vi "Setting_Screen.vi"(8 "error in (no error)":errorcluster) -> (0 "error in (out)":errorcluster)   [LabVIEW 2024, in "Setting_Screen.lvlib"]
doc: "This template is for the Queued Message Handler design pattern.\n\nThe Event Handling Loop generates messages based on user interface actions.\n\nThe Message Handling Loop processes messages generated by the Event Handling Loop, or by other messages. The messages are string values, so new messages can be added easily to the Message Cases case structure in the Message Handling Loop. Each message cluster can also provide an optional value for Message Data, which is a variant that can be converted to whatever message-specific data is required."
uses:
  Setting_Screen.lvlib
  support/Steptab.ctl
  support/PS_WRITE.ctl
  support/PS_set.ctl
  support/DMM_CONFIG.ctl
  support/READ_DATAS.ctl
  support/READ_EQP.ctl
  support/READ_PARA.ctl
  support/Relay_Channel_Array.ctl
  support/Common_plc_DOs.ctl
  support/DAQ_Config.ctl
  PCANusb_DTU/support/CAN_MSGs.ctl
  PCANusb_DTU/support/CAN_Frames_ctrl.ctl
  PCANusb_DTU/support/Framing datas.ctl
  PCANusb_DTU/support/CAN_Read.ctl
  support/Camera.ctl
  MCU_Flashing/support/MCU_ctrl.ctl
  support/Neoway ctl.ctl
  support/SSL.ctl
  controls/Setting_Screen UI Data.ctl
  support/ScriptDetails.ctl
  support/CurrentStep.ctl
  support/StepType.ctl
  PrivateControls/Setting_Screen_FGV_Queue_Control.ctl
  <vilib>/Utility/error.llb/Error Cluster From Error Code.vi
  <vilib>/ErrorRing/Error Ring.xnode
  support/Message Queue/Setting_Screen_Message Queue.lvlib
  support/User Event - Stop/Setting_Screen_User Event - Stop.lvlib
  Launcher/Launcher_DTU.lvlib
  Launcher/MainLauncher.vi
  PCANusb_DTU/PCANusb_DTU.lvlib
  MCU_Flashing/MCU_Flashing.lvlib
panel:
  out "Step no.":i16
  in  "New Step Name":string
  in  "Configurations:":string(combo)
  in  "Rename Step":bool
  in  "Instr.":bool
  in  "STEP_DOWN":bool
  in  "STEP_UP":bool
  in  "ADD NEXT SCRIPT":bool
  in  "SaveAs Name:":string
  in  "New_Config_name":string
  in  "New Config":bool
  in  "Save As":bool
  in  "Save":bool
  in  "UpdateStep":bool
  in  "Delete Step":bool
  in  "Delete Script":bool
  in  "Add Step":bool
  in  "Add Script":bool
  in  "Step Name":string
  in  "Script Name":string
  in  "Tab Control":T1
  in  "Set_Channel_Relay":T2 {"Relay_CH_Array"."OUTPUT_Relay_Channels" items=["CONN_SUPPLY_%d_FCT", "HB_CONN_%d_FCT", "L_IND_CONN_%d_FCT", "R_IND_CONN_%d_FCT", "SW1_%d_FCT", "SW2_%d_FCT", "CAN_H_%d_FCT", "CAN_L_%d_FCT", "CYLINDER_ON/OFF_%d_FCT", "SPARE_1_%d_FCT", "SPARE_2_%d_FCT", "Tower Red", "Tower Amber", "Tower Green", "Tower Buzzer", "SLIMRELAY_DUT_%d_FCT", "GND_DMM_%d_EOL", "CAN_H_RES_%d_EOL", "CAN_L_RES_%d_EOL", "L_IND_RES_%d_EOL", "R_IND_RES_%d_EOL", "HB_CONN_DMM_%d_EOL", "14V_RES_%d_EOL", "CAN_L_(DMM-)_%d_EOL", "CAN_H_%d_EOL", "CAN_L_%d_EOL", "14V_%d_EOL", "GND_%d_EOL", "HB_CONN_%d_EOL", "L_IND_%d_EOL", "R_IND_%d_EOL", "CYLINDER_DUT_%d_EOL", "CYL_PB_1_%d_EOL", "CYL_PB_2_%d_EOL", "DUT_PASS_%d_EOL", "DUT_FAIL_%d_EOL", "SPARE1_%d_EOL", "Tower Red_EOL", "Tower Amber_EOL", "Tower Green_EOL", "Tower Buzzer_EOL"]}
  in  "PS_Write":T4 {"Set_parameter" items=["Set_Voltage", "Set_current", "Output"]}
  in  "READ_DATAS":T6 {"PARAMETER" items=["SET_VOLTAGE", "SET_CURRENT", "OUTPUT VOLTAGE", "OUTPUT CURRENT", "RESISTANCE", "OUTPUT POWER", "CAMERA", "SSL_Check"]; "EQUIPMENT" items=["POWER SUPPLY", "DMM", "DAQ", "CAMERA"]}
  in  "DMM_CONFIG":T9 {"CONFIG PARAMETER" items=["VOLTAGE", "CURRENT", "RESISTANCE", "POWER"]}
  in  "DAQ_Config":T10 {"Function" items=["Voltage DC", "Voltage AC", "Current DC", "Current AC", "Resistance", "4-wire Resistance", "Diode", "Capacitance", "Temperature", "Continuity", "Frequency", "Period", "Voltage Ratio", "Digitize Voltage", "Digitize Current"]; "SELECT SLOT" items=["Slot 1", "Slot 2"]; "SELECT Card" items=["7708", "7700"]}
  in  "CAN_MSGs_Write":T11={"Scaling Factor"=1, "Physical value"=0.0, "CAN_Frames"={"CAN_ID"=0, "MSGTYPE"=128, "Payload"=[], "Length"=0}, "Offset value"=0.0, "Framing datas"=[], "CAN_Frame Enable"=FALSE, "Add Signal"=FALSE, "Delete Signal"=FALSE, "Signal Values"=[], "Time(ms)"=0.0, "Repetition"=FALSE, "Delay"=FALSE, "Delay time"=0.0} {"CAN_Frames"."Payload" format="%.0x"; "CAN_Frames"."MSGTYPE" items=["STATUS"=128, "EXTENDED"=2, "RTR"=1, "DATA MSG"=0]; "CAN_Frames"."CAN_ID" format="%.0x"}
  in  "CAN_Read":T14 {"SUB-SERVICE ID" format="%.0x"; "SERVICE ID" format="%.0x"; "CANID" format="%.0x"; "ReadPayload" format="%.0x"}
  in  "Camera":T15
  in  "Noeway_Flashing":T16
  in  "MCU Flashing":T17
  in  "SSL":T18
  in  "Script_Tree":string(tree)
  out "queue name 2":string
  out "queue name":string
  in  "New Step":bool
  in  "New Script":bool
  in  "Exit":bool
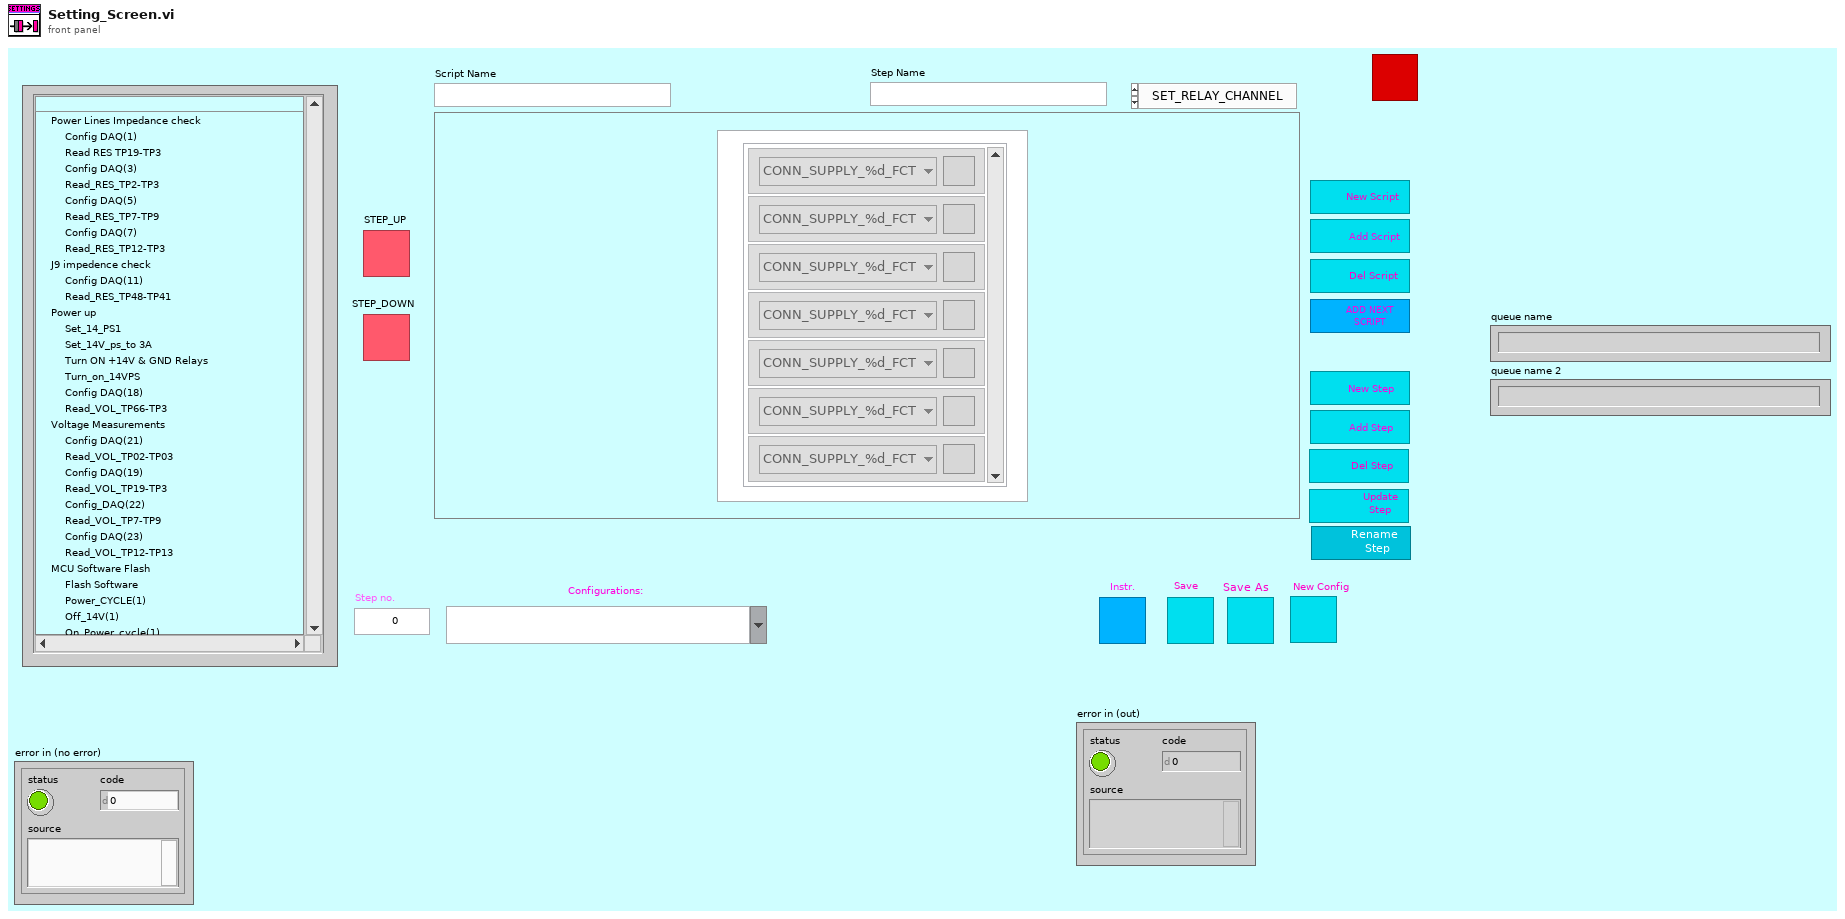
[diagram p1: front panel]
types:
  T1 = typedef "Setting_Screen.lvlib/Steptab.ctl" = enum32{"SET_RELAY_CHANNEL", "PS_WRITE", "READ_DATA", "DMM_CONFIG", "DAQ_Config", "CAN_Write", "CAN_Read", "Camera", "Noeway_Flashing", "MCU_Flashing", "SSL_Certification"}
  T2 = typedef "Setting_Screen.lvlib/Relay_Channel_Array.ctl" = cluster{"Relay_CH_Array":cluster{"OUTPUT_Relay_Channels":T3, "On/Off":bool}[]}
  T3 = typedef "Setting_Screen.lvlib/Common_plc_DOs.ctl" = u16
  T4 = typedef "Setting_Screen.lvlib/PS_WRITE.ctl" = cluster{"Set_parameter":T5, "VOLTAGE":string, "CURRENT":string, "OUTPUT":bool, "Delay":bool, "Delay time":dbl}
  T5 = typedef "Setting_Screen.lvlib/PS_set.ctl" = u16
  T6 = typedef "Setting_Screen.lvlib/READ_DATAS.ctl" = cluster{"EQUIPMENT":T7, "PARAMETER":T8, "LSL":dbl, "USL":dbl, "RESULT":string, "UNIT":string, "Delay":bool, "Delay time":dbl}
  T7 = typedef "Setting_Screen.lvlib/READ_EQP.ctl" = u16
  T8 = typedef "Setting_Screen.lvlib/READ_PARA.ctl" = u16
  T9 = typedef "Setting_Screen.lvlib/DMM_CONFIG.ctl" = cluster{"CONFIG PARAMETER":u16, "AUTO RANGE":bool, "RANGE":string, "Delay":bool, "Delay time":dbl}
  T10 = typedef "Setting_Screen.lvlib/DAQ_Config.ctl" = cluster{"AUTO RANGE":bool, "CHANNEL LIST":string, "SELECT Card":u16, "SELECT SLOT":u16, "Function":i32}
  T11 = typedef "PCANusb_DTU.lvlib/CAN_MSGs.ctl" = cluster{"Scaling Factor":u16, "Physical value":dbl, "CAN_Frames":T12, "Offset value":dbl, "Framing datas":T13[], "CAN_Frame Enable":bool, "Add Signal":bool, "Delete Signal":bool, "Signal Values":dbl[], "Time(ms)":dbl, "Repetition":bool, "Delay":bool, "Delay time":dbl}
  T12 = typedef "PCANusb_DTU.lvlib/CAN_Frames_ctrl.ctl" = cluster{"CAN_ID":u32, "MSGTYPE":u8, "Payload":u8[], "Length":u8}
  T13 = typedef "PCANusb_DTU.lvlib/Framing datas.ctl" = cluster{"Signal name":string, "Start Bit":u8, "Length":u8, "Value":u16}
  T14 = typedef "PCANusb_DTU.lvlib/CAN_Read.ctl" = cluster{"Database":refnum<k21>, "Signal":refnum<k21>, "BYTES":u32[], "ReadPayload":u8[], "String_Data":string, "ReadValue":dbl, "CANID":u32, "SERVICE ID":u32, "SUB-SERVICE ID":u32, "DELAY ":bool, "Delay time(ms)":dbl}
  T15 = typedef "Setting_Screen.lvlib/Camera.ctl" = cluster{"Trigger":bool, "Prog No.":string, "Delay":bool, "Delay time":dbl, "Storage":string, "Col no.":string, "Row no.":string}
  T16 = typedef "Neoway ctl.ctl" = cluster{"Neoway_Firmware":path, "RESULT STRING":string, "Delay":bool, "Delay time":dbl}
  T17 = typedef "MCU_Flashing.lvlib/MCU_ctrl.ctl" = cluster{"Result Path":path, "Result":string}
  T18 = typedef "SSL.ctl" = cluster{"SSL_EXE":path, "RESULT STRING":string, "Delay":bool, "Delay time":dbl}
  T19 = typedef "Setting_Screen.lvlib/Setting_Screen_FGV_Queue_Control.ctl" = enum16{"Release", "Get", "Set"}
  T20 = typedef "Setting_Screen.lvlib/Setting_Screen UI Data.ctl" = cluster{"Script_Tree":refnum<vi>, "Scripts":T21[], "ScriptDetails":T21, "Current Step":T22, "ScriptName":string, "StepName":string, "Children Symbols":i32[][], "Parrent Symbol":i32[], "Configurations:":string, "Config":string, "Scriptno.":i32, "PS_Write":T4, "DMM_CONFIG":T9, "READ_DATAS":T6, "Set_Channel_Relay":T2, "DAQ_Config":T10, "CAN_MSGs_Write":T11, "CAN_Read":T14, "Camera":T15, "Tab Control":refnum<vi>, "MCU Flashing":T17, "Noeway_Flashing":T16, "SSL":T18}
  T21 = typedef "Setting_Screen.lvlib/ScriptDetails.ctl" = cluster{"Script Name":string, "Steps":T22[]}
  T22 = typedef "Setting_Screen.lvlib/CurrentStep.ctl" = cluster{"StepName":string, "StepDetails":string, "Type":T23}
  T23 = typedef "Setting_Screen.lvlib/StepType.ctl" = enum16{"RELAY_CHANNEL_WRITE", "PS_WRITE", "READ_DATA", "DMM_CONFIG", "DAQ_CONFIG", "PCAN_Read", "PCAN_Write", "Camera", "MCU_Flashing", "Noeway_Flashing", "SSL_Certification"}
  T24 = typedef "Setting_Screen.lvlib/Setting_Screen_Message Queue.lvlib/Setting_ScreenAll Message Queues.ctl" = cluster{"UI":refnum<queue>, "QSM":refnum<queue>}
  T25 = enum16{"Next Item", "Previous Item", "Get Child", "Get Parent", "Get Path"}
  T26 = enum16{"Read", "Write", "All_sections", "All_values", "Remove key&section"}
  T27 = enum32{"Invalid", "Standard", "Closed", "Hidden", "Minimized", "Maximized"}
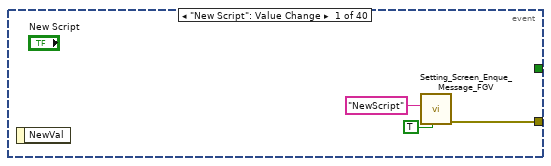
[diagram p3: hidden frame]
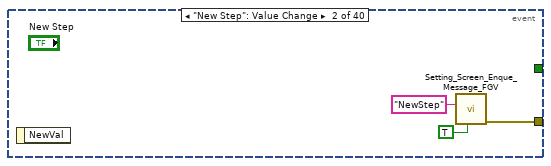
[diagram p4: hidden frame]
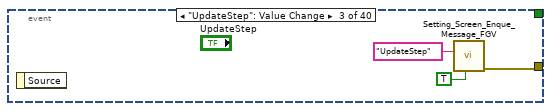
[diagram p5: hidden frame]
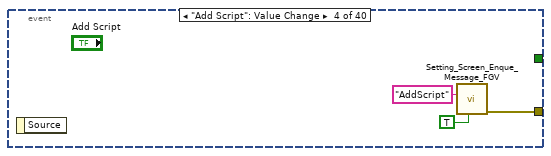
[diagram p6: hidden frame]
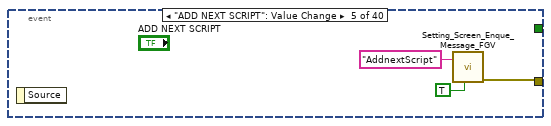
[diagram p7: hidden frame]
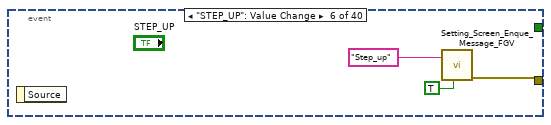
[diagram p8: hidden frame]
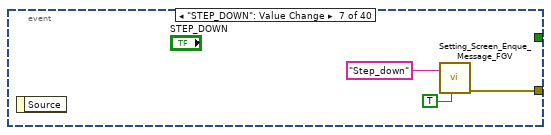
[diagram p9: hidden frame]
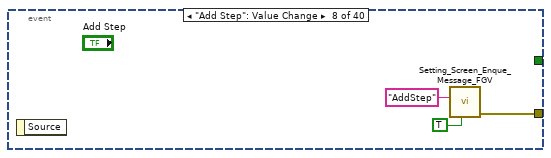
[diagram p10: hidden frame]
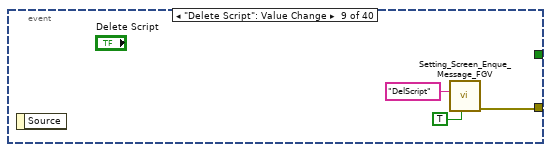
[diagram p11: hidden frame]
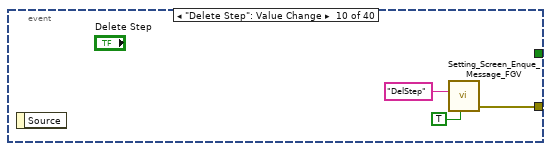
[diagram p12: hidden frame]
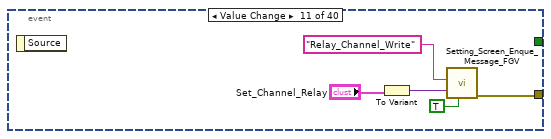
[diagram p13: hidden frame]
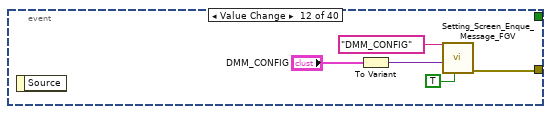
[diagram p14: hidden frame]
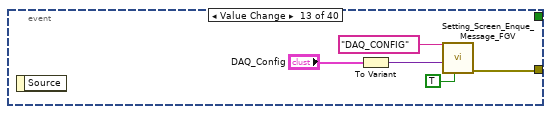
[diagram p15: hidden frame]
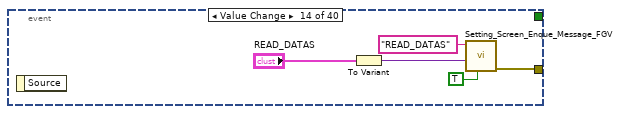
[diagram p16: hidden frame]
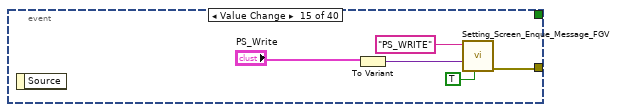
[diagram p17: hidden frame]
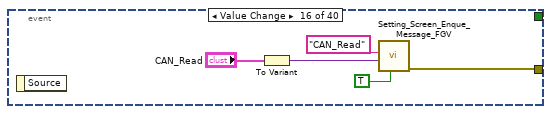
[diagram p18: hidden frame]
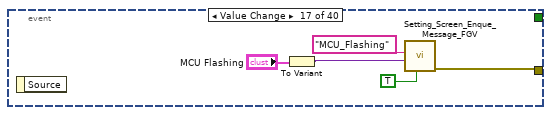
[diagram p19: hidden frame]
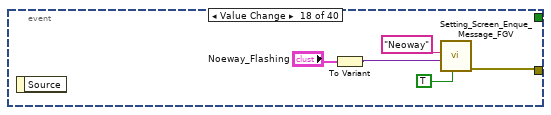
[diagram p20: hidden frame]
diagram:
  (unwired) 40
  (unwired) "\u0000\u0000\u0000\u0000\u0000\u0000\u0000\u000f\u0000\u0000\u0000\u0000\u0000\u0000\u0000\u0001\u0000\u0000\u0000\u0000\u0000\u0000\u0000\u0000\u0000\u0000\u0000\u0000\u0000#Signal connector J9 impedence check\u0000\u0000\u0000\u0016\u0000\u0000\u0000\u000eConfig_DMM_RES\u0000\u0000\u0000\u0010\u0000\u0002\u0001\u0000\u0000\u0000\u0000\u0000\u0000\u0000\u0000\u0000\u0000\u0000\u0000\u0000\u0000\u0003\u0000\u0000\u0000\u001aTurn ON CAN_H & GND Relays\u0000\u0000\u0000\n\u0000\u0000\u0000\u0002\u0000\u0010\u0001\u0000\u0011\u0001\u0000\u0000\u0000\u0000\u0000\u0015Read RES CAN_H to GND\u0000\u0000\u0000)\u0000\u0001\u0000\u0004?ð\u0000\u0000\u0000\u0000\u0000\u0000@$\u0000\u0000\u0000\u0000\u0000\u0000\u0000\u0000\u0000\u0000\u0000\u0000\u0000\u0004Mohm\u0000\u0000\u0000\u0000\u0000\u0000\u0000\u0000\u0000\u0000\u0002\u0000\u0000\u0000\u0015Turn OFF CAN _H Relay\u0000\u0000\u0000\u0007\u0000\u0000\u0000\u0001\u0000\u0011\u0000\u0000\u0000\u0000\u0000\u0000\u0013Turn ON CAN_L Relay\u0000\u0000\u0000\u0007\u0000\u0000\u0000\u0001\u0000\u0012\u0001\u0000\u0000\u0000\u0000\u0000\u0015Read RES CAN_L to GND\u0000\u0000\u0000)\u0000\u0001\u0000\u0004?ð\u0000\u0000\u0000\u0000\u0000\u0000@$\u0000\u0000\u0000\u0000\u0000\u0000\u0000\u0000\u0000\u0000\u0000\u0000\u0000\u0004Mohm\u0000\u0000\u0000\u0000\u0000\u0000\u0000\u0000\u0000\u0000\u0002\u0000\u0000\u0000\u001bTurn OFF CAN_L & GND Relays\u0000\u0000\u0000\n\u0000\u0000\u0000\u0002\u0000\u0010\u0000\u0000\u0012\u0000\u0000\u0000\u0000\u0000\u0000\u001cTurn ON CAN_H & CAN_L Relays\u0000\u0000\u0000\n\u0000\u0000\u0000\u0002\u0000\u0011\u0001\u0000\u0017\u0001\u0000\u0000\u0000\u0000\u0000\u0016Read RES CAN_H & CAN_L\u0000\u0000\u0000(\u0000\u0001\u0000\u0004@]\u0000\u0000\u0000\u0000\u0000@^\u0000\u0000\u0000\u0000\u0000\u0000\u0000\u0000\u0000\u0000\u0000\u0000\u0003ohm\u0000\u0000\u0000\u0000\u0000\u0000\u0000\u0000\u0000\u0000\u0002\u0000\u0000\u0000\u001dTurn OFF CAN_H & CAN_L Relays\u0000\u0000\u0000\n\u0000\u0000\u0000\u0002\u0000\u0011\u0000\u0000\u0017\u0000\u0000\u0000\u0000\u0000\u0000\u001aTurn ON..." ("data string")
  w20 = T20 {"Script_Tree"=refnum, "Scripts"=[], "ScriptDetails"={"Script Name"="", "Steps"=[]}, "Current Step"={"StepName"="", "StepDetails"="", "Type"=enum."RELAY_CHANNEL_WRITE"}, "ScriptName"="", "StepName"="", "Children Symbols"=[], "Parrent Symbol"=[], "Configurations:"="", "Config"="", "Scriptno."=0, "PS_Write"={"Set_parameter"=0, "VOLTAGE"="", "CURRENT"="", "OUTPUT"=FALSE, "Delay"=FALSE, "Delay time"=0.0}, "DMM_CONFIG"={"CONFIG PARAMETER"=0, "AUTO RANGE"=FALSE, "RANGE"="", "Delay"=FALSE, "Delay time"=0.0}, "READ_DATAS"={"EQUIPMENT"=0, "PARAMETER"=0, "LSL"=0.0, "USL"=0.0, "RESULT"="", "UNIT"="", "Delay"=FALSE, "Delay time"=0.0}, "Set_Channel_Relay"={"Relay_CH_Array"=[]}, "DAQ_Config"={"AUTO RANGE"=FALSE, "CHANNEL LIST"="", "SELECT Card"=0, "SELECT SLOT"=0, "Function"=0}, "CAN_MSGs_Write"={"Scaling Factor"=0, "Physical value"=0.0, "CAN_Frames"={"CAN_ID"=0, "MSGTYPE"=0, "Payload"=[], "Length"=0}, "Offset value"=0.0, "Framing datas"=[], "CAN_Frame Enable"=FALSE, "Add Signal"=FALSE, "Delete Signal"=FALSE, "Signal Values"=[], "Time(ms)"=0.0, "Repetition"=FALSE, "Delay"=FALSE, "Delay time"=0.0}, "CAN_Read"={"Database"="", "Signal"="", "BYTES"=[], "ReadPayload"=[], "String_Data"="", "ReadValue"=0.0, "CANID"=0, "SERVICE ID"=0, "SUB-SERVICE ID"=0, "DELAY "=FALSE, "Delay time(ms)"=0.0}, "Camera"={"Trigger"=FALSE, "Prog No."="", "Delay"=FALSE, "Delay time"=0.0, "Storage"="", "Col no."="", "Row no."=""}, "Tab Control"=refnum, "MCU Flashing"={"Result Path"=path "", "Result"=""}, "Noeway_Flashing"={"Neoway_Firmware"=path "", "RESULT STRING"="", "Delay"=FALSE, "Delay time"=0.0}, "SSL"={"SSL_EXE"=path "", "RESULT STRING"="", "Delay"=FALSE, "Delay time"=0.0}}  # Data Cluster
  # "MCU_Flashing"
  n1 = control-ref of="This VI"() -> (w15:refnum<vi>)
  n2 = call "Setting_Screen_Pre_Loop_Initialization_FGV.vi"("error in (no error)"="error in (no error)", "VI in"=w15) -> ("error out"=w13:errorcluster, "User Event out"=w4:refnum<user-event>)  [unwired: 8 in]
  n3 = call "Create User Event - Stop.vi"("error in (no error)"=w13) -> ("error out"=w8:errorcluster, "User Event - Stop"=w3:refnum<user-event>)  [unwired: 9 in]
  n4 = control-ref of="This VI"() -> (w11:refnum<vi>)
  n5 = register-events(w3, w4) -> (reference out=w18:refnum<event-registration>, error out=w16:errorcluster)  [unwired: 2 in]
  n6 = call "Setting_Screen_Create All Message Queues.vi"("error in (no error)"=w8, "This VI"=w11) -> ("error out"=w27:errorcluster, "Message Queues out"=w26:T24)  [unwired: 8 in]
  n7 = Unbundle By Name(w26) -> ("UI"=w24:refnum<queue>)
  n8 = call "Setting_Screen_Queue_Comm_FGV.vi"("error in (no error)"=w8, "Enum"=Setting_Screen_FGV_Queue_Control."Get") -> ("queue Out"=w6:refnum<queue>)  [unwired: 8 in, 1 out]
  n9 = Get Queue Status(queue=w24) -> (queue out=w10:refnum<queue>, queue name=→"queue name":string)  [unwired: 2 in, 6 out]
  n10 = Get Queue Status(queue=w6) -> (queue name=→"queue name 2":string)  [unwired: 2 in, 7 out]
  n11 = Merge Errors(w16, w27) -> (w17:errorcluster)
  n12 = while {
    tunnel: w10 -> [_]
    shift-right: [w37] -> _
    shift-left: w20 -> [w38]
    tunnel: w4 -> [w35]
    tunnel: w17 -> [w34]
    tunnel: [w29] -> w25
    tunnel: w3 -> [w28]
    stop <- w36 stop-if-true
    # "Message Handling Loop FGV"
    n13 = call "Setting_Screen_Dequeue_Message_FGV.vi"("error in (no error)"=w34) -> ("error out"=w33:errorcluster, "Message Data"=w32:variant, "Message"=w31:string)  [unwired: 8 in]
    n14 = case "Message Cases" shown="\"AddnextScript\"" w31 {
      selector: w31 -> [_ _ _ _ _ _ _ _ _ _ _ _ _ _ _ _ _ _ _ _ _ _ _ _ _ _ _ _ _ _ _ _ _ _ _ _ _ _ _ _ _ _ _ _ _ w918]
      tunnel: w33 -> [w55 w83 w129 w144 w170 w189 w199 w207 w222 w249 w272 w292 w312 w345 w374 w386 w417 w453 w470 w483 w496 w509 w522 w535 w548 w561 w578 w604 w607 w614 w629 w642 w654 w778 w813 w819 w844 w851 w860 w867 w874 w890 w898 w901 w909 _]
      tunnel: [w66 w75 w107 w135 w169 w194 w204 w206 w220 w247 w268 w290 w310 w343 w373 w384 w415 w452 w470 w480 w492 w505 w518 w531 w544 w557 w566 w600 w608 w613 w628 w641 w653 w761 w795 w818 w843 w850 w859 w865 w872 w891 w892 w903 w915 w919] -> w30
      tunnel: w38 -> [w68 w85 w126 w133 w183 w195 w205 w210 w217 w244 w271 w285 w307 w340 w375 w381 w412 w450 w469 w478 w489 w502 w515 w528 w541 w554 w573 w597 w611 w619 w627 w640 w650 w777 w812 w820 w845 w852 w858 w866 w873 w889 w897 w904 w917 w920]
      tunnel: [w67 w85 w118 w139 w175 w187 w197 w210 w216 w243 w270 w284 w306 w338 w375 w380 w411 w444 w468 w481 w493 w506 w519 w532 w545 w558 w575 w601 w609 w617 w626 w639 w649 w758 w792 w820 w840 w852 w858 w862 w869 w889 w897 w904 w917 w920] -> w37
      tunnel: [_ _ _ _ _ _ _ _ _ _ _ _ _ _ _ _ _ _ _ _ _ _ _ _ _ _ _ _ _ _ _ _ _ _ _ _ _ _ _ _ _ _ _ _ TRUE _] -> w36
      tunnel: w32 -> [_ _ w103 w143 _ _ _ _ _ _ _ _ _ w336 _ _ _ _ _ w473 w494 w507 w520 w533 w546 w559 w576 w602 _ _ w624 w637 _ _ w783 _ w841 _ _ w863 w870 _ w896 _ w911 _]
      tunnel: w35 -> [_ _ _ _ _ _ _ _ _ _ _ _ _ _ _ _ _ _ _ _ _ _ _ _ _ _ _ _ _ _ _ _ _ _ _ _ _ _ _ _ _ _ _ _ w914 _]
      tunnel: w28 -> [_ _ _ _ _ _ _ _ _ _ _ _ _ _ _ _ _ _ _ _ _ _ _ _ _ _ _ _ _ _ _ _ _ _ _ _ _ _ _ _ _ _ _ _ w907 _]
      frame "Initialize" {
        w40 = T2 {"Relay_CH_Array"=[{"OUTPUT_Relay_Channels"=0, "On/Off"=FALSE}]}  # Set_Channel_Relay
        w43 = T9 {"CONFIG PARAMETER"=0, "AUTO RANGE"=FALSE, "RANGE"="", "Delay"=FALSE, "Delay time"=0.0}  # DMM_CONFIG
        w44 = T6 {"EQUIPMENT"=0, "PARAMETER"=0, "LSL"=0.0, "USL"=0.0, "RESULT"="", "UNIT"="", "Delay"=FALSE, "Delay time"=0.0}  # READ_DATAS
        w45 = T4 {"Set_parameter"=0, "VOLTAGE"="", "CURRENT"="", "OUTPUT"=FALSE, "Delay"=FALSE, "Delay time"=0.0}  # PS_Write
        w56 = ""
        w60 = ""
        w62 = T22 {"StepName"="", "StepDetails"="", "Type"=enum."RELAY_CHANNEL_WRITE"}  # Current Step
        w63 = T21 {"Script Name"="", "Steps"=[]}  # ScriptDetails
        w64 = T21[] [{"Script Name"="", "Steps"=[{"StepName"="", "StepDetails"="", "Type"=enum."RELAY_CHANNEL_WRITE"}]}]  # Scripts
        # "Initialize"
        n15 = control-ref of="Script_Tree"() -> (w54:refnum<vi>)
        n16 = property on="SaveAs Name:" class="Str"("Visible"=FALSE, "Value"="" ("SaveAs Name:")) -> ()  [unwired: 2 in, 2 out]
        n17 = property on="New Step Name" class="Str"("Visible"=FALSE, "Value"="" ("New Step Name")) -> ()  [unwired: 2 in, 2 out]
        n18 = property class="Tree (strict)"(reference=w54, error in=w55) -> (reference out=w52:refnum<vi>, error out=w53:errorcluster, "All Tags"=w51:string[])
        n19 = property on="New_Config_name" class="Str"("Value"="" ("New_Config_name"), "Visible"=FALSE) -> ()  [unwired: 2 in, 2 out]
        n20 = property on="Configurations:" class="CmbBox"("Strings[]"=string[] [] ("Strings []")) -> ()  [unwired: 2 in, 2 out]
        n21 = for {
          tunnel: w52 -> [w73]
          tunnel: w51 -> [w72] mode=indexing
          shift-right: [w69] -> w50
          shift-left: w53 -> [w74]
          n22 = invoke class="Tree (strict)" method="Edit Tree Items.Delete"(reference=w73, error in=w74, "tag"=w72, "Delete Children"=TRUE ("Delete Children?")) -> (error out=w70:errorcluster)  [unwired: 1 in, 4 out]
          n23 = call <vilib>:"Clear Errors.vi"("error in (no error)"=w70) -> ("error out"=w69:errorcluster)  [unwired: 5 in, 1 out]
        }
        n24 = control-ref of="Script_Tree"() -> (w61:refnum<vi>)
        n25 = control-ref of="Tab Control"() -> (w39:refnum<vi>)
        n26 = Bundle By Name(cluster=w68, "DMM_CONFIG"=w43, "READ_DATAS"=w44, "Scriptno."=0, "Script_Tree"=w61, "Tab Control"=w39, "PS_Write"=w45, "Set_Channel_Relay"=w40, "Scripts"=w64, "ScriptDetails"=w63, "Current Step"=w62, "ScriptName"=w60, "StepName"=w60, "Config"=w60, "Configurations:"="") -> (w67:T20)
        n27 = local write "Script_Tree"(w56) -> ()
        n28 = property class="Tree (strict)"(reference=w61, "Value"=w56) -> ()  [unwired: 1 in, 2 out]
        n29 = call "Setting_Screen_Enque_Message_FGV.vi"("error in (no error)"=w50, "Message"="ReadConfig") -> ("error out"=w66:errorcluster)  [unwired: 9 in]
      }
      frame "ReadConfig" {
        n30 = call "Specify_Path.vi"("Path_Enum"=enum16{"Find_Path", "Get_Path"}."Get_Path", "error in (no error)"=w83) -> ("Settings"=w78:path, "error out"=w82:errorcluster)  [unwired: 6 in, 6 out]
        n31 = List Folder(path=w78, error in=w82) -> (filenames=w79:string[], error out=w81:errorcluster)  [unwired: 2 in, 2 out]
        n32 = Empty Array?(array=w79) -> (empty?=w80:bool)
        n33 = case shown="False" w80 {
          tunnel: w81 -> [w90 w96]
          tunnel: [w90 w96] -> w76
          tunnel: w79 -> [w88 _]
          tunnel: w78 -> [w89 _]
          frame False {
            n34 = for {
              tunnel: w89 -> [w93]
              tunnel: w88 -> [w92] mode=indexing
              tunnel: [w91] -> w87 mode=indexing
              n35 = Build Path(base path=w93, name or relative path=w92) -> (appended path=w94:path)
              n36 = call <vilib>:"Get File Extension.vi"("file"=w94) -> ("filename without extension"=w91:string)  [unwired: 6 in, 4 out]
            }
            n37 = property on="Configurations:" class="CmbBox"("Strings[]"=w87, "Value"="" ("Configurations:")) -> ()  [unwired: 2 in, 2 out]
          }
          frame True {
            n38 = property on="New_Config_name" class="Str"("Visible"=TRUE) -> ()  [unwired: 2 in, 2 out]
          }
        }
        n39 = call "Setting_Screen_Enque_Message_FGV.vi"("error in (no error)"=w76, "Message"="Update Display") -> ("error out"=w75:errorcluster)  [unwired: 9 in]
      }
      frame "ReadSelected" {
        n40 = Variant To Data(error in=w129, type="" ("Configurations:"), Variant=w103) -> (data=w99:string, error out=w104:errorcluster)
        n41 = Unbundle By Name(w126) -> ("Configurations:"=w100:string)
        n42 = call <vilib>:"Clear Errors.vi"("error in (no error)"=w104) -> ("error out"=w98:errorcluster)  [unwired: 5 in, 1 out]
        n43 = Empty String/Path?(string/path=w99) -> (empty?=w101:bool)
        n44 = call "Specify_Path.vi"("Path_Enum"=enum16{"Find_Path", "Get_Path"}."Get_Path", "error in (no error)"=w98) -> ("Settings"=w105:path, "error out"=w128:errorcluster)  [unwired: 6 in, 6 out]
        n45 = Select(t=w100, s=w101, f=w99) -> (s? t:f=w97:string)
        n46 = Concatenate Strings(w97, ".bin" ("string")) -> (w125:string)
        n47 = Build Path(base path=w105, name or relative path=w125) -> (appended path=w122:path)
        n48 = call "BIN_File.vi"("Enum"=enum16{"Read", "Write"}."Read", "error in"=w128, "Path"=w122) -> ("error out"=w123:errorcluster, "data out"=w120:string)  [unwired: 7 in]
        n49 = Unflatten From String(type=T20 {"Script_Tree"=refnum, "Scripts"=[], "ScriptDetails"={"Script Name"="", "Steps"=[]}, "Current Step"={"StepName"="", "StepDetails"="", "Type"=enum."RELAY_CHANNEL_WRITE"}, "ScriptName"="", "StepName"="", "Children Symbols"=[], "Parrent Symbol"=[], "Configurations:"="", "Config"="", "Scriptno."=0, "PS_Write"={"Set_parameter"=0, "VOLTAGE"="", "CURRENT"="", "OUTPUT"=FALSE, "Delay"=FALSE, "Delay time"=0.0}, "DMM_CONFIG"={"CONFIG PARAMETER"=0, "AUTO RANGE"=FALSE, "RANGE"="", "Delay"=FALSE, "Delay time"=0.0}, "READ_DATAS"={"EQUIPMENT"=0, "PARAMETER"=0, "LSL"=0.0, "USL"=0.0, "RESULT"="", "UNIT"="", "Delay"=FALSE, "Delay time"=0.0}, "Set_Channel_Relay"={"Relay_CH_Array"=[]}, "DAQ_Config"={"AUTO RANGE"=FALSE, "CHANNEL LIST"="", "SELECT Card"=0, "SELECT SLOT"=0, "Function"=0}, "CAN_MSGs_Write"={"Scaling Factor"=0, "Physical value"=0.0, "CAN_Frames"={"CAN_ID"=0, "MSGTYPE"=0, "Payload"=[], "Length"=0}, "Offset value"=0.0, "Framing datas"=[], "CAN_Frame Enable"=FALSE, "Add Signal"=FALSE, "Delete Signal"=FALSE, "Signal Values"=[], "Time(ms)"=0.0, "Repetition"=FALSE, "Delay"=FALSE, "Delay time"=0.0}, "CAN_Read"={"Database"="", "Signal"="", "BYTES"=[], "ReadPayload"=[], "String_Data"="", "ReadValue"=0.0, "CANID"=0, "SERVICE ID"=0, "SUB-SERVICE ID"=0, "DELAY "=FALSE, "Delay time(ms)"=0.0}, "Camera"={"Trigger"=FALSE, "Prog No."="", "Delay"=FALSE, "Delay time"=0.0, "Storage"="", "Col no."="", "Row no."=""}, "Tab Control"=refnum, "MCU Flashing"={"Result Path"=path "", "Result"=""}, "Noeway_Flashing"={"Neoway_Firmware"=path "", "RESULT STRING"="", "Delay"=FALSE, "Delay time"=0.0}, "SSL"={"SSL_EXE"=path "", "RESULT STRING"="", "Delay"=FALSE, "Delay time"=0.0}} ("Data Cluster"), binary string=w120, error in (no error)=w123) -> (value=w117:T20, error out=w109:errorcluster)  [unwired: 2 in, 1 out]
        n50 = Unbundle By Name(w117) -> ("Script_Tree"=w116:refnum<vi>, "Scripts"=w115:T21[], "Children Symbols"=w114:i32[][], "Parrent Symbol"=w113:i32[], "Tab Control"=w112:refnum<vi>)
        n51 = Bundle By Name(cluster=w126, "Configurations:"=w97, "Script_Tree"=w116, "Scripts"=w115, "Children Symbols"=w114, "Parrent Symbol"=w113, "Tab Control"=w112) -> (w118:T20)
        n52 = call "Setting_Screen_Queue_Comm_FGV.vi"("error in (no error)"=w109, "Enum"=Setting_Screen_FGV_Queue_Control."Get") -> ("error Out"=w108:errorcluster, "queue Out"=w111:refnum<queue>)  [unwired: 8 in]
        n53 = call "Setting_Screen_Enqueue Message (Array).vi"("error in (no error)"=w108, "Message Array"=string[] ["DrawTree", "Update Display"], "Message Queue"=w111) -> ("error out"=w107:errorcluster)  [unwired: 7 in, 1 out]
      }
      frame "ScriptTree" {
        n54 = Variant To Data(error in=w144, type="" ("Script_Tree"), Variant=w143) -> (data=w138:string, error out=w141:errorcluster)
        n55 = Empty String/Path?(string/path=w138) -> (empty?=w140:bool)
        n56 = case shown="False" w140 {
          tunnel: w141 -> [w166 w167]
          tunnel: [w165 w167] -> w136
          tunnel: w138 -> [w163 _]
          tunnel: [w161 _] -> w137
          frame False {
            n57 = control-ref of="Script_Tree"() -> (w164:refnum<vi>)
            n58 = call "Tree_navigation.vi"("error in (no error)"=w166, "Tag"=w163, "Operation"=T25."Get Parent", "Script_Tree"=w164) -> ("error out"=w165:errorcluster, "Data"=w161:string)  [unwired: 5 in, 1 out]
          }
          frame True {
          }
        }
        n59 = Unbundle By Name(w133) -> ("Scripts"=w132:T21[])
        n60 = Empty String/Path?(string/path=w137) -> (empty?=w134:bool)
        n61 = Select(t=w138, s=w134, f=w137) -> (s? t:f=w131:string)
        n62 = case shown="True" w134 {
          tunnel: w136 -> [w149 w158]
          tunnel: [w147 w156] -> w135
          tunnel: w132 -> [_ w154]
          tunnel: w131 -> [_ w153]
          tunnel: [0 ("Script") w152] -> w130
          frame False {
            n63 = call "Setting_Screen_Queue_Comm_FGV.vi"("error in (no error)"=w149, "Enum"=Setting_Screen_FGV_Queue_Control."Get") -> ("error Out"=w148:errorcluster, "queue Out"=w151:refnum<queue>)  [unwired: 8 in]
            n64 = call "Setting_Screen_Enqueue Message (Array).vi"("error in (no error)"=w148, "Message Array"=string[] ["Get_Step", "Update Display"], "Message Queue"=w151) -> ("error out"=w147:errorcluster)  [unwired: 7 in, 1 out]
          }
          frame True {
            n65 = call "GetStep.vi"("Parent (Script)"=w153, "Scripts"=w154) -> ("Script"=w152:i32)  [unwired: 7 in, 2 out]
            n66 = call "Setting_Screen_Queue_Comm_FGV.vi"("error in (no error)"=w158, "Enum"=Setting_Screen_FGV_Queue_Control."Get") -> ("error Out"=w157:errorcluster, "queue Out"=w160:refnum<queue>)  [unwired: 8 in]
            n67 = call "Setting_Screen_Enqueue Message (Array).vi"("error in (no error)"=w157, "Message Array"=string[] ["Update Display"], "Message Queue"=w160) -> ("error out"=w156:errorcluster)  [unwired: 7 in, 1 out]
          }
        }
        n68 = Bundle By Name(cluster=w133, "StepName"=w138, "ScriptName"=w131, "Scriptno."=w130) -> (w139:T20)
      }
      frame "En/Dis_Script" {
        n69 = Unbundle By Name(w183) -> ("Scripts"=w179:T21[], "Parrent Symbol"=w178:i32[], "Scriptno."=w177:i32)
        n70 = Index Array(array=w178, index=w177) -> (element=w182:i32)
        n71 = Equal?(x=w182, y=40) -> (x = y?=w180:bool)
        n72 = case shown="False" w180 {
          tunnel: [40 37] -> w176
          frame False {
          }
          frame True {
          }
        }
        n73 = Replace Array Subset(array=w178, new element=w176, index=w177) -> (w174:i32[])
        n74 = Bundle By Name(cluster=w183, "Scripts"=w179, "Parrent Symbol"=w174) -> (w175:T20)
        n75 = call "Setting_Screen_Queue_Comm_FGV.vi"("error in (no error)"=w170, "Enum"=Setting_Screen_FGV_Queue_Control."Get") -> ("error Out"=w173:errorcluster, "queue Out"=w172:refnum<queue>)  [unwired: 8 in]
        n76 = call "Setting_Screen_Enqueue Message (Array).vi"("error in (no error)"=w173, "Message Array"=string[] ["DrawTree", "Update Display"], "Message Queue"=w172) -> ("error out"=w169:errorcluster)  [unwired: 7 in, 1 out]
      }
      frame "NewScript" {
        # "New Script involvement"
        n77 = Bundle By Name(cluster=w195, "ScriptName"="") -> (w187:T20)
        n78 = call "Setting_Screen_Queue_Comm_FGV.vi"("error in (no error)"=w189, "Enum"=Setting_Screen_FGV_Queue_Control."Get") -> ("error Out"=w191:errorcluster, "queue Out"=w193:refnum<queue>)  [unwired: 8 in]
        n79 = call "Setting_Screen_Enqueue Message (Array).vi"("error in (no error)"=w191, "Message Array"=string[] ["Reset Step", "Update Display"], "Message Queue"=w193) -> ("error out"=w188:errorcluster)  [unwired: 7 in, 1 out]
        n80 = Merge Errors(w188) -> (w194:errorcluster)
      }
      frame "NewStep" {
        # "New Step Involvement"
        n81 = Bundle By Name(cluster=w205, "StepName"="") -> (w197:T20)
        n82 = call "Setting_Screen_Queue_Comm_FGV.vi"("error in (no error)"=w199, "Enum"=Setting_Screen_FGV_Queue_Control."Get") -> ("error Out"=w201:errorcluster, "queue Out"=w203:refnum<queue>)  [unwired: 8 in]
        n83 = call "Setting_Screen_Enqueue Message (Array).vi"("error in (no error)"=w201, "Message Array"=string[] ["Reset Step", "Update Display"], "Message Queue"=w203) -> ("error out"=w198:errorcluster)  [unwired: 7 in, 1 out]
        n84 = Merge Errors(w198) -> (w204:errorcluster)
      }
      frame "UpdateStep" {
        n85 = call "Setting_Screen_Enque_Message_FGV.vi"("error in (no error)"=w207, "Message Data"="UpdateStep" ("Initial Message"), "Message"="AddStep") -> ("error out"=w206:errorcluster)  [unwired: 8 in]
      }
      frame "AddScript" {
        n86 = Unbundle By Name(w217) -> ("Scripts"=w214:T21[], "ScriptName"=w213:string, "Parrent Symbol"=w212:i32[])
        n87 = call "GetStep.vi"("Parent (Script)"=w213, "Scripts"=w214) -> ("Script"=w215:i32)  [unwired: 7 in, 2 out]
        n88 = case shown="-1" w215 {
          tunnel: w217 -> [w224 w236]
          tunnel: [w224 w235] -> w216
          tunnel: w214 -> [_ w234]
          tunnel: w213 -> [_ w231]
          tunnel: w212 -> [_ w228]
          tunnel: [string[] ["Update Display"] ("Message Array") string[] ["Reset Step", "DrawTree", "Update Display"] ("Message Array")] -> w211
          frame 0, Default {
          }
          frame -1 {
            n89 = Bundle By Name(cluster=T21 {"Script Name"="", "Steps"=[]} ("ScriptDetails"), "Script Name"=w231) -> (w230:T21)
            n90 = Build Array (concatenate)(w228, 40) -> (w227:i32[])
            n91 = Build Array (concatenate)(w234, w230) -> (w233:T21[])
            n92 = Bundle By Name(cluster=w236, "ScriptName"="", "Scripts"=w233, "Parrent Symbol"=w227) -> (w235:T20)
          }
        }
        n93 = call "Setting_Screen_Queue_Comm_FGV.vi"("error in (no error)"=w222, "Enum"=Setting_Screen_FGV_Queue_Control."Get") -> ("error Out"=w221:errorcluster, "queue Out"=w219:refnum<queue>)  [unwired: 8 in]
        n94 = call "Setting_Screen_Enqueue Message (Array).vi"("error in (no error)"=w221, "Message Array"=w211, "Message Queue"=w219) -> ("error out"=w220:errorcluster)  [unwired: 7 in, 1 out]
      }
      frame "AddnextScript" {
        n95 = Unbundle By Name(w244) -> ("Scriptno."=w237:i32, "Scripts"=w241:T21[], "ScriptName"=w240:string, "Parrent Symbol"=w239:i32[])
        n96 = call "GetStep.vi"("Parent (Script)"=w240, "Scripts"=w241) -> ("Script"=w242:i32)  [unwired: 7 in, 2 out]
        n97 = case shown="-1" w242 {
          tunnel: w244 -> [w251 w265]
          tunnel: [w251 w264] -> w243
          tunnel: w241 -> [_ w263]
          tunnel: w240 -> [_ w260]
          tunnel: w239 -> [_ w255]
          tunnel: [string[] ["Update Display"] ("Message Array") string[] ["Reset Step", "DrawTree", "Update Display"] ("Message Array")] -> w238
          tunnel: w237 -> [_ w257]
          frame 0, Default {
          }
          frame -1 {
            n98 = Increment(x=w257) -> (x+1=w254:i32)
            n99 = Bundle By Name(cluster=T21 {"Script Name"="", "Steps"=[]} ("ScriptDetails"), "Script Name"=w260) -> (w256:T21)
            n100 = Insert Into Array(array=w255, index=w254, new element=40) -> (w252:i32[])
            n101 = Insert Into Array(array=w263, index=w254, new element=w256) -> (w262:T21[])
            n102 = Bundle By Name(cluster=w265, "ScriptName"="", "Scripts"=w262, "Parrent Symbol"=w252) -> (w264:T20)
          }
        }
        n103 = call "Setting_Screen_Queue_Comm_FGV.vi"("error in (no error)"=w249, "Enum"=Setting_Screen_FGV_Queue_Control."Get") -> ("error Out"=w248:errorcluster, "queue Out"=w246:refnum<queue>)  [unwired: 8 in]
        n104 = call "Setting_Screen_Enqueue Message (Array).vi"("error in (no error)"=w248, "Message Array"=w238, "Message Queue"=w246) -> ("error out"=w247:errorcluster)  [unwired: 7 in, 1 out]
      }
      frame "AddStep" {
        n105 = call "Add.vi"("error in"=w272, "UI Data"=w271) -> ("error out"=w269:errorcluster, "Draw"=w266:bool, "Valid"=w267:bool, "UI Data out"=w270:T20)  [unwired: 6 in]
        n106 = case shown="True" w267 {
          tunnel: w269 -> [w273 w280]
          tunnel: [w273 w278] -> w268
          tunnel: w266 -> [_ w274]
          frame False {
          }
          frame True {
            n107 = Select(t=string[] ["Reset Step", "DrawTree", "Update Display"], s=w274, f=string[] ["Update Display"]) -> (s? t:f=w275:string[])
            n108 = call "Setting_Screen_Queue_Comm_FGV.vi"("error in (no error)"=w280, "Enum"=Setting_Screen_FGV_Queue_Control."Get") -> ("error Out"=w279:errorcluster, "queue Out"=w282:refnum<queue>)  [unwired: 8 in]
            n109 = call "Setting_Screen_Enqueue Message (Array).vi"("error in (no error)"=w279, "Message Array"=w275, "Message Queue"=w282) -> ("error out"=w278:errorcluster)  [unwired: 7 in, 1 out]
          }
        }
      }
      frame "DelScript" {
        n110 = Unbundle By Name(w285) -> ("Scripts"=w287:T21[], "ScriptName"=w289:string, "Parrent Symbol"=w286:i32[])
        n111 = call "GetStep.vi"("Parent (Script)"=w289, "Scripts"=w287) -> ("Script"=w288:i32)  [unwired: 7 in, 2 out]
        n112 = case shown="0, Default" w288 {
          selector: w288 -> [w300 _]
          tunnel: w287 -> [w303 _]
          tunnel: w286 -> [w302 _]
          tunnel: w285 -> [w297 w304]
          tunnel: [w296 w304] -> w284
          tunnel: [string[] ["Reset Step", "DrawTree", "Update Display"] string[] ["Update Display"]] -> w283
          frame 0, Default {
            w301 = 1 ("length")
            n113 = Delete From Array(array=w303, length=w301, index=w300) -> (array with subset deleted=w299:T21[])  [unwired: 1 out]
            n114 = Delete From Array(array=w302, length=w301, index=w300) -> (array with subset deleted=w298:i32[])  [unwired: 1 out]
            n115 = Bundle By Name(cluster=w297, "Scripts"=w299, "Parrent Symbol"=w298) -> (w296:T20)
          }
          frame -1 {
          }
        }
        n116 = call "Setting_Screen_Queue_Comm_FGV.vi"("error in (no error)"=w292, "Enum"=Setting_Screen_FGV_Queue_Control."Get") -> ("error Out"=w291:errorcluster, "queue Out"=w294:refnum<queue>)  [unwired: 8 in]
        n117 = call "Setting_Screen_Enqueue Message (Array).vi"("error in (no error)"=w291, "Message Array"=w283, "Message Queue"=w294) -> ("error out"=w290:errorcluster)  [unwired: 7 in, 1 out]
      }
      frame "DelStep" {
        # "Delete Step"
        n118 = Unbundle By Name(w307) -> ("Scripts"=w308:T21[], "ScriptName"=w318:string, "StepName"=w317:string)
        n119 = call "GetStep.vi"("Child (Step)"=w317, "Parent (Script)"=w318, "Scripts"=w308) -> ("Step"=w316:i32, "Script"=w315:i32)  [unwired: 6 in, 1 out]
        n120 = case shown="0, Default" w316 {
          selector: w316 -> [w322 _]
          tunnel: w315 -> [w325 _]
          tunnel: [string[] ["DrawTree", "Reset Step", "Update Display"] string[] ["Update Display"]] -> w309
          tunnel: w308 -> [w323 _]
          tunnel: w307 -> [w320 w332]
          tunnel: [w319 w332] -> w306
          frame 0, Default {
            n121 = in-place {
              in-place-border: w322 -> [w326]
              n122 = in-place-array #1(w323, w325) -> (w330:T21)
              n123 = Unbundle By Name(w330) -> ("Steps"=w331:T22[])
              n124 = Delete From Array(array=w331, length=1, index=w326) -> (array with subset deleted=w329:T22[])  [unwired: 1 out]
              n125 = Bundle By Name(cluster=w330, "Steps"=w329) -> (w328:T21)
              n126 = in-place-array #1(w328) -> (w321:T21[])  [unwired: 1 out]
            }
            n127 = Bundle By Name(cluster=w320, "Scripts"=w321) -> (w319:T20)
          }
          frame -1 {
          }
        }
        n128 = call "Setting_Screen_Queue_Comm_FGV.vi"("error in (no error)"=w312, "Enum"=Setting_Screen_FGV_Queue_Control."Get") -> ("error Out"=w311:errorcluster, "queue Out"=w314:refnum<queue>)  [unwired: 8 in]
        n129 = call "Setting_Screen_Enqueue Message (Array).vi"("error in (no error)"=w311, "Message Array"=w309, "Message Queue"=w314) -> ("error out"=w310:errorcluster)  [unwired: 7 in, 1 out]
      }
      frame "NewStepname" {
        # "NewStepname"
        n130 = Variant To Data(error in=w345, type="", Variant=w336) -> (data=w334:string, error out=w337:errorcluster)
        n131 = Unbundle By Name(w340) -> ("Scripts"=w341:T21[], "ScriptName"=w351:string, "StepName"=w350:string)
        n132 = call "GetStep.vi"("Child (Step)"=w350, "Parent (Script)"=w351, "Scripts"=w341) -> ("Step"=w349:i32, "Script"=w348:i32)  [unwired: 6 in, 1 out]
        n133 = case shown="0, Default" w349 {
          selector: w349 -> [w359 _]
          tunnel: w348 -> [w362 _]
          tunnel: [string[] ["DrawTree", "Reset Step", "Update Display"] string[] ["Update Display"]] -> w342
          tunnel: w341 -> [w360 _]
          tunnel: w340 -> [w357 w371]
          tunnel: [w356 w371] -> w339
          tunnel: w334 -> [w355 _]
          frame 0, Default {
            n134 = in-place {
              in-place-border: w359 -> [w363]
              in-place-border: w355 -> [w364]
              n135 = in-place-array #2(w360, w362) -> (w370:T21)
              n136 = Unbundle By Name(w370) -> ("Steps"=w366:T22[])
              n137 = Index Array(array=w366, index=w363) -> (element=w368:T22)
              n138 = Bundle By Name(cluster=w368, "StepName"=w364) -> (w367:T22)
              n139 = Replace Array Subset(array=w366, new element=w367, index=w363) -> (w365:T22[])
              n140 = Bundle By Name(cluster=w370, "Steps"=w365) -> (w369:T21)
              n141 = in-place-array #2(w369) -> (w358:T21[])  [unwired: 1 out]
            }
            n142 = Bundle By Name(cluster=w357, "Scripts"=w358) -> (w356:T20)
          }
          frame -1 {
          }
        }
        n143 = flat-sequence {
          tunnel: [w353] -> w338
          tunnel: w339 -> [w353]
          frame #0 {
            n144 = property on="New Step Name" class="Str"("Visible"=FALSE, "Value"="" ("New Step Name")) -> ()  [unwired: 2 in, 2 out]
          }
        }
        n145 = call "Setting_Screen_Queue_Comm_FGV.vi"("error in (no error)"=w337, "Enum"=Setting_Screen_FGV_Queue_Control."Get") -> ("error Out"=w344:errorcluster, "queue Out"=w347:refnum<queue>)  [unwired: 8 in]
        n146 = call "Setting_Screen_Enqueue Message (Array).vi"("error in (no error)"=w344, "Message Array"=w342, "Message Queue"=w347) -> ("error out"=w343:errorcluster)  [unwired: 7 in, 1 out]
      }
      frame "Rename_Step" {
        n147 = flat-sequence {
          tunnel: w374 -> [w379]
          tunnel: [w378] -> w373
          frame #0 {
            n148 = property on="New Step Name" class="Str"(error in=w379, "Visible"=TRUE, "Value"="" ("New Step Name")) -> (error out=w378:errorcluster)  [unwired: 1 in, 1 out]
          }
        }
      }
      frame "Step_up" {
        # "Move one step upwards or before"
        n149 = Unbundle By Name(w381) -> ("Scripts"=w382:T21[], "ScriptName"=w392:string, "StepName"=w391:string)
        n150 = call "GetStep.vi"("Child (Step)"=w391, "Parent (Script)"=w392, "Scripts"=w382) -> ("Step"=w390:i32, "Script"=w389:i32)  [unwired: 6 in, 1 out]
        n151 = case shown="0, Default" w390 {
          selector: w390 -> [w396 _]
          tunnel: w389 -> [w399 _]
          tunnel: [string[] ["DrawTree", "Update Display"] string[] ["Update Display"]] -> w383
          tunnel: w382 -> [w397 _]
          tunnel: w381 -> [w394 w409]
          tunnel: [w393 w409] -> w380
          frame 0, Default {
            n152 = in-place {
              in-place-border: w396 -> [w404]
              n153 = in-place-array #3(w397, w399) -> (w408:T21)
              n154 = Unbundle By Name(w408) -> ("Steps"=w405:T22[])
              n155 = Index Array(array=w405, index=w404) -> (element=w401:T22)
              n156 = Delete From Array(array=w405, length=1, index=w404) -> (array with subset deleted=w403:T22[])  [unwired: 1 out]
              n157 = Decrement(x=w404) -> (x-1=w402:i32)
              n158 = Insert Into Array(array=w403, index=w402, new element=w401) -> (w400:T22[])
              n159 = Bundle By Name(cluster=w408, "Steps"=w400) -> (w407:T21)
              n160 = in-place-array #3(w407) -> (w395:T21[])  [unwired: 1 out]
            }
            n161 = Bundle By Name(cluster=w394, "Scripts"=w395) -> (w393:T20)
          }
          frame -1 {
          }
        }
        n162 = call "Setting_Screen_Queue_Comm_FGV.vi"("error in (no error)"=w386, "Enum"=Setting_Screen_FGV_Queue_Control."Get") -> ("error Out"=w385:errorcluster, "queue Out"=w388:refnum<queue>)  [unwired: 8 in]
        n163 = call "Setting_Screen_Enqueue Message (Array).vi"("error in (no error)"=w385, "Message Array"=w383, "Message Queue"=w388) -> ("error out"=w384:errorcluster)  [unwired: 7 in, 1 out]
      }
      frame "Step_down" {
        # "Move one step down or afterwards"
        n164 = Unbundle By Name(w412) -> ("Scripts"=w413:T21[], "ScriptName"=w423:string, "StepName"=w422:string)
        n165 = call "GetStep.vi"("Child (Step)"=w422, "Parent (Script)"=w423, "Scripts"=w413) -> ("Step"=w421:i32, "Script"=w420:i32)  [unwired: 6 in, 1 out]
        n166 = case shown="0, Default" w421 {
          selector: w421 -> [w427 _]
          tunnel: w420 -> [w430 _]
          tunnel: [string[] ["DrawTree", "Update Display"] string[] ["Update Display"]] -> w414
          tunnel: w413 -> [w428 _]
          tunnel: w412 -> [w425 w440]
          tunnel: [w424 w440] -> w411
          frame 0, Default {
            n167 = in-place {
              in-place-border: w427 -> [w435]
              n168 = in-place-array #4(w428, w430) -> (w439:T21)
              n169 = Unbundle By Name(w439) -> ("Steps"=w436:T22[])
              n170 = Index Array(array=w436, index=w435) -> (element=w432:T22)
              n171 = Delete From Array(array=w436, length=1, index=w435) -> (array with subset deleted=w434:T22[])  [unwired: 1 out]
              n172 = Increment(x=w435) -> (x+1=w433:i32)
              n173 = Insert Into Array(array=w434, index=w433, new element=w432) -> (w431:T22[])
              n174 = Bundle By Name(cluster=w439, "Steps"=w431) -> (w438:T21)
              n175 = in-place-array #4(w438) -> (w426:T21[])  [unwired: 1 out]
            }
            n176 = Bundle By Name(cluster=w425, "Scripts"=w426) -> (w424:T20)
          }
          frame -1 {
          }
        }
        n177 = call "Setting_Screen_Queue_Comm_FGV.vi"("error in (no error)"=w417, "Enum"=Setting_Screen_FGV_Queue_Control."Get") -> ("error Out"=w416:errorcluster, "queue Out"=w419:refnum<queue>)  [unwired: 8 in]
        n178 = call "Setting_Screen_Enqueue Message (Array).vi"("error in (no error)"=w416, "Message Array"=w414, "Message Queue"=w419) -> ("error out"=w415:errorcluster)  [unwired: 7 in, 1 out]
      }
      frame "DrawTree" {
        n179 = Unbundle By Name(w450) -> ("Children Symbols"=w445:i32[][], "Parrent Symbol"=w446:i32[], "Scripts"=w449:T21[])  [unwired: 1 out]
        n180 = control-ref of="Script_Tree"() -> (w442:refnum<vi>)
        n181 = for {
          tunnel: w449 -> [w457] mode=indexing
          tunnel: [w455] -> w448 mode=indexing
          tunnel: [w454] -> w447 mode=indexing
          n182 = Unbundle By Name(w457) -> ("Script Name"=w454:string, "Steps"=w456:T22[])
          n183 = for {
            tunnel: w456 -> [w459] mode=indexing
            tunnel: [w458] -> w455 mode=indexing
            n184 = Unbundle By Name(w459) -> ("StepName"=w458:string)
          }
        }
        n185 = call "Empty_tree.vi"("error in (no error)"=w453, "Script_Tree"=w442) -> ("error out"=w451:errorcluster)  [unwired: 8 in, 1 out]
        n186 = call "Add_tree.vi"("Children Symbols"=w445, "Parrent Symbol"=w446, "error in"=w451, "Children"=w448, "Parent"=w447, "Script_Tree"=w442) -> ("error IO"=w452:errorcluster, "Script_Treeout"=w443:refnum<vi>)  [unwired: 4 in]
        n187 = Bundle By Name(cluster=w450, "Script_Tree"=w443) -> (w444:T20)
      }
      frame "Reset Step" {
        w465 = T6 {"EQUIPMENT"=0, "PARAMETER"=0, "LSL"=0.0, "USL"=0.0, "RESULT"="", "UNIT"="", "Delay"=FALSE, "Delay time"=0.0}  # READ_DATAS
        w466 = T9 {"CONFIG PARAMETER"=0, "AUTO RANGE"=FALSE, "RANGE"="", "Delay"=FALSE, "Delay time"=0.0}  # DMM_CONFIG
        w467 = T4 {"Set_parameter"=0, "VOLTAGE"="", "CURRENT"="", "OUTPUT"=FALSE, "Delay"=FALSE, "Delay time"=0.0}  # PS_Write
        n188 = Bundle By Name(cluster=w469, "Set_Channel_Relay"=T2 {"Relay_CH_Array"=[]}, "PS_Write"=w467, "DMM_CONFIG"=w466, "READ_DATAS"=w465, "DAQ_Config"=T10 {"AUTO RANGE"=FALSE, "CHANNEL LIST"="", "SELECT Card"=0, "SELECT SLOT"=0, "Function"=0}, "CAN_MSGs_Write"=T11 {"Scaling Factor"=1, "Physical value"=0.0, "CAN_Frames"={"CAN_ID"=0, "MSGTYPE"=128, "Payload"=[], "Length"=0}, "Offset value"=0.0, "Framing datas"=[], "CAN_Frame Enable"=FALSE, "Add Signal"=FALSE, "Delete Signal"=FALSE, "Signal Values"=[], "Time(ms)"=0.0, "Repetition"=FALSE, "Delay"=FALSE, "Delay time"=0.0}, "CAN_Read"=T14 {"Database"="", "Signal"="", "BYTES"=[], "ReadPayload"=[], "String_Data"="", "ReadValue"=0.0, "CANID"=0, "SERVICE ID"=0, "SUB-SERVICE ID"=0, "DELAY "=FALSE, "Delay time(ms)"=0.0}, "Camera"=T15 {"Trigger"=FALSE, "Prog No."="", "Delay"=FALSE, "Delay time"=0.0, "Storage"="", "Col no."="", "Row no."=""}) -> (w468:T20)
      }
      frame "Relay_Channel_Write" {
        w472 = T2 {"Relay_CH_Array"=[]}  # Set_Channel_Relay
        w479 = T22 {"StepName"="", "StepDetails"="", "Type"=enum."RELAY_CHANNEL_WRITE"}  # Current Step
        n189 = Variant To Data(error in=w483, type=w472, Variant=w473) -> (data=w471:T2, error out=w482:errorcluster)
        n190 = Unbundle By Name(w478) -> ("StepName"=w477:string)
        n191 = Flatten To String(anything=w471, error in (no error)=w482) -> (data string=w475:string, error out=w480:errorcluster)  [unwired: 2 in, 1 out]
        n192 = Bundle By Name(cluster=w479, "StepName"=w477, "Type"=StepType."RELAY_CHANNEL_WRITE", "StepDetails"=w475) -> (w476:T22)
        n193 = Bundle By Name(cluster=w478, "Current Step"=w476, "Set_Channel_Relay"=w471) -> (w481:T20)
      }
      frame "DMM_CONFIG" {
        w490 = T22 {"StepName"="", "StepDetails"="", "Type"=enum."RELAY_CHANNEL_WRITE"}  # Current Step
        n194 = Variant To Data(error in=w496, type=T9 {"CONFIG PARAMETER"=0, "AUTO RANGE"=FALSE, "RANGE"="", "Delay"=FALSE, "Delay time"=0.0} ("DMM_CONFIG"), Variant=w494) -> (data=w491:T9, error out=w495:errorcluster)
        n195 = Unbundle By Name(w489) -> ("StepName"=w488:string)
        n196 = Flatten To String(anything=w491, error in (no error)=w495) -> (data string=w487:string, error out=w492:errorcluster)  [unwired: 2 in, 1 out]
        n197 = Bundle By Name(cluster=w490, "StepName"=w488, "Type"=StepType."DMM_CONFIG", "StepDetails"=w487) -> (w486:T22)
        n198 = Bundle By Name(cluster=w489, "Current Step"=w486, "DMM_CONFIG"=w491) -> (w493:T20)
      }
      frame "DAQ_CONFIG" {
        w503 = T22 {"StepName"="", "StepDetails"="", "Type"=enum."RELAY_CHANNEL_WRITE"}  # Current Step
        n199 = Variant To Data(error in=w509, type=T10 {"AUTO RANGE"=FALSE, "CHANNEL LIST"="", "SELECT Card"=0, "SELECT SLOT"=0, "Function"=0} ("DAQ_Config"), Variant=w507) -> (data=w504:T10, error out=w508:errorcluster)
        n200 = Unbundle By Name(w502) -> ("StepName"=w501:string)
        n201 = Flatten To String(anything=w504, error in (no error)=w508) -> (data string=w500:string, error out=w505:errorcluster)  [unwired: 2 in, 1 out]
        n202 = Bundle By Name(cluster=w503, "StepName"=w501, "Type"=StepType."DAQ_CONFIG", "StepDetails"=w500) -> (w499:T22)
        n203 = Bundle By Name(cluster=w502, "Current Step"=w499, "DAQ_Config"=w504) -> (w506:T20)
      }
      frame "READ_DATAS" {
        w516 = T22 {"StepName"="", "StepDetails"="", "Type"=enum."RELAY_CHANNEL_WRITE"}  # Current Step
        n204 = Variant To Data(error in=w522, type=T6 {"EQUIPMENT"=0, "PARAMETER"=0, "LSL"=0.0, "USL"=0.0, "RESULT"="", "UNIT"="", "Delay"=FALSE, "Delay time"=0.0} ("READ_DATAS"), Variant=w520) -> (data=w517:T6, error out=w521:errorcluster)
        n205 = Unbundle By Name(w515) -> ("StepName"=w514:string)
        n206 = Flatten To String(anything=w517, error in (no error)=w521) -> (data string=w513:string, error out=w518:errorcluster)  [unwired: 2 in, 1 out]
        n207 = Bundle By Name(cluster=w516, "StepName"=w514, "Type"=StepType."READ_DATA", "StepDetails"=w513) -> (w512:T22)
        n208 = Bundle By Name(cluster=w515, "Current Step"=w512, "READ_DATAS"=w517) -> (w519:T20)
      }
      frame "CAN_Read" {
        w529 = T22 {"StepName"="", "StepDetails"="", "Type"=enum."RELAY_CHANNEL_WRITE"}  # Current Step
        n209 = Variant To Data(error in=w535, type=T14 {"Database"="", "Signal"="", "BYTES"=[], "ReadPayload"=[], "String_Data"="", "ReadValue"=0.0, "CANID"=0, "SERVICE ID"=0, "SUB-SERVICE ID"=0, "DELAY "=FALSE, "Delay time(ms)"=0.0} ("CAN_Read"), Variant=w533) -> (data=w530:T14, error out=w534:errorcluster)
        n210 = Unbundle By Name(w528) -> ("StepName"=w527:string)
        n211 = Flatten To String(anything=w530, error in (no error)=w534) -> (data string=w526:string, error out=w531:errorcluster)  [unwired: 2 in, 1 out]
        n212 = Bundle By Name(cluster=w529, "StepName"=w527, "Type"=StepType."PCAN_Read", "StepDetails"=w526) -> (w525:T22)
        n213 = Bundle By Name(cluster=w528, "Current Step"=w525, "CAN_Read"=w530) -> (w532:T20)
      }
      frame "MCU_Flashing" {
        w542 = T22 {"StepName"="", "StepDetails"="", "Type"=enum."RELAY_CHANNEL_WRITE"}  # Current Step
        n214 = Variant To Data(error in=w548, type=T17 {"Result Path"=path "", "Result"=""} ("MCU Flashing"), Variant=w546) -> (data=w543:T17, error out=w547:errorcluster)
        n215 = Unbundle By Name(w541) -> ("StepName"=w540:string)
        n216 = Flatten To String(anything=w543, error in (no error)=w547) -> (data string=w539:string, error out=w544:errorcluster)  [unwired: 2 in, 1 out]
        n217 = Bundle By Name(cluster=w542, "StepName"=w540, "Type"=StepType."MCU_Flashing", "StepDetails"=w539) -> (w538:T22)
        n218 = Bundle By Name(cluster=w541, "Current Step"=w538, "MCU Flashing"=w543) -> (w545:T20)
      }
      frame "SSL" {
        w555 = T22 {"StepName"="", "StepDetails"="", "Type"=enum."RELAY_CHANNEL_WRITE"}  # Current Step
        n219 = Variant To Data(error in=w561, type=T18 {"SSL_EXE"=path "", "RESULT STRING"="", "Delay"=FALSE, "Delay time"=0.0} ("SSL"), Variant=w559) -> (data=w556:T18, error out=w560:errorcluster)
        n220 = Unbundle By Name(w554) -> ("StepName"=w553:string)
        n221 = Flatten To String(anything=w556, error in (no error)=w560) -> (data string=w552:string, error out=w557:errorcluster)  [unwired: 2 in, 1 out]
        n222 = Bundle By Name(cluster=w555, "StepName"=w553, "Type"=StepType."SSL_Certification", "StepDetails"=w552) -> (w551:T22)
        n223 = Bundle By Name(cluster=w554, "Current Step"=w551, "SSL"=w556) -> (w558:T20)
      }
      frame "Neoway" {
        w574 = T22 {"StepName"="", "StepDetails"="", "Type"=enum."RELAY_CHANNEL_WRITE"}  # Current Step
        n224 = Variant To Data(error in=w578, type=T16 {"Neoway_Firmware"=path "", "RESULT STRING"="", "Delay"=FALSE, "Delay time"=0.0} ("Noeway_Flashing"), Variant=w576) -> (data=w565:T16, error out=w577:errorcluster)
        n225 = Unbundle By Name(w573) -> ("StepName"=w572:string)
        n226 = Unbundle By Name(w565) -> ("Neoway_Firmware"=w564:path)
        n227 = Flatten To String(anything=w565, error in (no error)=w577) -> (data string=w571:string, error out=w567:errorcluster)  [unwired: 2 in, 1 out]
        n228 = Bundle By Name(cluster=w574, "StepName"=w572, "Type"=StepType."Noeway_Flashing", "StepDetails"=w571) -> (w570:T22)
        n229 = Path To String(path=w564) -> (string=w563:string)
        n230 = Build Array(w563) -> (w562:string[])
        n231 = Bundle By Name(cluster=w573, "Current Step"=w570, "Noeway_Flashing"=w565) -> (w575:T20)
        n232 = disable-structure shown="Disabled" {
          disable-tunnel: w567 -> [w582 _]
          disable-tunnel: [w581 _] -> w566
          disable-tunnel: w562 -> [w579 _]
          frame Disabled {
            n233 = call "Specify_Path.vi"("Path_Enum"=enum16{"Find_Path", "Get_Path"}."Get_Path", "error in (no error)"=w582) -> ("Configurations"=w583:path, "error out"=w587:errorcluster)  [unwired: 6 in, 6 out]
            n234 = Concatenate Strings("Flash_Paths" ("string"), ".ini" ("string")) -> (w589:string)
            n235 = Build Path(base path=w583, name or relative path=w589) -> (appended path=w588:path)
            n236 = call "INI_driver.vi"("Enum"=T26."Write", "instrument file path"=w588, "error in (no error)"=w587, "Value_in"=w579, "Section"="Neoway", "Key_name"=string[] ["PAC_FILE"]) -> ("error out"=w581:errorcluster)  [unwired: 2 in, 3 out]
          }
          frame Enabled {
          }
        }
      }
      frame "CAN_Write" {
        w598 = T22 {"StepName"="", "StepDetails"="", "Type"=enum."RELAY_CHANNEL_WRITE"}  # Current Step
        n237 = Variant To Data(error in=w604, type=T11 {"Scaling Factor"=0, "Physical value"=128.0, "CAN_Frames"={"CAN_ID"=0, "MSGTYPE"=128, "Payload"=[], "Length"=0}, "Offset value"=0.0, "Framing datas"=[], "CAN_Frame Enable"=FALSE, "Add Signal"=FALSE, "Delete Signal"=FALSE, "Signal Values"=[], "Time(ms)"=0.0, "Repetition"=FALSE, "Delay"=FALSE, "Delay time"=0.0} ("CAN_MSGs_Write"), Variant=w602) -> (data=w599:T11, error out=w603:errorcluster)
        n238 = Unbundle By Name(w597) -> ("StepName"=w596:string)
        n239 = Flatten To String(anything=w599, error in (no error)=w603) -> (data string=w595:string, error out=w600:errorcluster)  [unwired: 2 in, 1 out]
        n240 = Bundle By Name(cluster=w598, "StepName"=w596, "Type"=StepType."PCAN_Write", "StepDetails"=w595) -> (w594:T22)
        n241 = Bundle By Name(cluster=w597, "Current Step"=w594, "CAN_MSGs_Write"=w599) -> (w601:T20)
      }
      frame "Add_Signal" {
        n242 = Unbundle By Name(w611) -> ("CAN_MSGs_Write"=w612:T11)
        n243 = call "Add_Signal.vi"("CAN_MSGs"=w612) -> ("CAN_MSGs 2"=w610:T11)  [unwired: 10 in]
        n244 = Bundle By Name(cluster=w611, "CAN_MSGs_Write"=w610) -> (w609:T20)
        n245 = call "Enque_Message_FGV.vi"("error in (no error)"=w607, "Message Data"="Add_Signal" ("Message"), "Message"="Update Display") -> ("error out"=w608:errorcluster)  [unwired: 8 in]
      }
      frame "Delete_Signal" {
        n246 = Unbundle By Name(w619) -> ("CAN_MSGs_Write"=w620:T11)
        n247 = call "Delete_Signal.vi"("CAN_MSGs"=w620) -> ("CAN_MSGs 2"=w618:T11)  [unwired: 10 in]
        n248 = Bundle By Name(cluster=w619, "CAN_MSGs_Write"=w618) -> (w617:T20)
        n249 = call "Enque_Message_FGV.vi"("error in (no error)"=w614, "Message Data"="Delete_Signal" ("Message"), "Message"="Update Display") -> ("error out"=w613:errorcluster)  [unwired: 8 in]
      }
      frame "PS_WRITE" {
        w632 = T22 {"StepName"="", "StepDetails"="", "Type"=enum."RELAY_CHANNEL_WRITE"}  # Current Step
        n250 = Unbundle By Name(w627) -> ("StepName"=w631:string)
        n251 = Variant To Data(error in=w629, type=T4 {"Set_parameter"=0, "VOLTAGE"="", "CURRENT"="", "OUTPUT"=FALSE, "Delay"=FALSE, "Delay time"=0.0} ("PS_Write"), Variant=w624) -> (data=w623:T4, error out=w633:errorcluster)
        n252 = Flatten To String(anything=w623, error in (no error)=w633) -> (data string=w630:string, error out=w628:errorcluster)  [unwired: 2 in, 1 out]
        n253 = Bundle By Name(cluster=w632, "StepName"=w631, "Type"=StepType."PS_WRITE", "StepDetails"=w630) -> (w625:T22)
        n254 = Bundle By Name(cluster=w627, "Current Step"=w625, "PS_Write"=w623) -> (w626:T20)
      }
      frame "Camera" {
        w645 = T22 {"StepName"="", "StepDetails"="", "Type"=enum."RELAY_CHANNEL_WRITE"}  # Current Step
        n255 = Unbundle By Name(w640) -> ("StepName"=w644:string)
        n256 = Variant To Data(error in=w642, type=T15 {"Trigger"=FALSE, "Prog No."="", "Delay"=FALSE, "Delay time"=0.0, "Storage"="", "Col no."="", "Row no."=""} ("Camera"), Variant=w637) -> (data=w636:T15, error out=w646:errorcluster)
        n257 = Flatten To String(anything=w636, error in (no error)=w646) -> (data string=w643:string, error out=w641:errorcluster)  [unwired: 2 in, 1 out]
        n258 = Bundle By Name(cluster=w645, "StepName"=w644, "Type"=StepType."Camera", "StepDetails"=w643) -> (w638:T22)
        n259 = Bundle By Name(cluster=w640, "Current Step"=w638, "Camera"=w636) -> (w639:T20)
      }
      frame "Get_Step" {
        n260 = Unbundle By Name(w650) -> ("Scripts"=w659:T21[], "ScriptName"=w661:string, "StepName"=w660:string)
        n261 = call "GetStep.vi"("Child (Step)"=w660, "Parent (Script)"=w661, "Scripts"=w659) -> ("Step"=w647:i32, "Script"=w658:i32)  [unwired: 6 in, 1 out]
        "Step no." <- w647
        n262 = Index Array(array=w659, index=w658) -> (element=w657:T21)
        n263 = Unbundle By Name(w657) -> ("Steps"=w656:T22[])
        n264 = Index Array(array=w656, index=w647) -> (element=w655:T22)
        n265 = Unbundle By Name(w655) -> ("StepName"=w648:string, "Type"=w652:T23, "StepDetails"=w651:string)
        n266 = case shown="\"RELAY_CHANNEL_WRITE\", Default" w652 {
          tunnel: w654 -> [w669 w677 w685 w693 w701 w709 w717 w725 w733 w741 w749]
          tunnel: [w668 w676 w684 w692 w700 w708 w716 w724 w731 w735 w743] -> w653
          tunnel: w651 -> [w667 w675 w683 w691 w699 w707 w715 w723 w732 w740 w748]
          tunnel: w650 -> [w666 w673 w681 w689 w697 w705 w713 w721 w729 w739 w747]
          tunnel: [w665 w671 w680 w688 w696 w704 w712 w720 w727 w738 w746] -> w649
          tunnel: w648 -> [_ _ _ _ _ _ _ _ _ _ _]
          frame "RELAY_CHANNEL_WRITE", Default {
            n267 = Unbundle By Name(w666) -> ("Set_Channel_Relay"=w663:T2)
            n268 = Unflatten From String(type=w663, binary string=w667, error in (no error)=w669) -> (value=w662:T2, error out=w668:errorcluster)  [unwired: 2 in, 1 out]
            n269 = Bundle By Name(cluster=w666, "Set_Channel_Relay"=w662) -> (w665:T20)
            n270 = property on="Tab Control" class="TabCtl (strict)"("Value"=Steptab."SET_RELAY_CHANNEL" ("Tab Control")) -> ()  [unwired: 2 in, 2 out]
          }
          frame "PS_WRITE" {
            n271 = Unbundle By Name(w673) -> ("PS_Write"=w674:T4)
            n272 = Unflatten From String(type=w674, binary string=w675, error in (no error)=w677) -> (value=w672:T4, error out=w676:errorcluster)  [unwired: 2 in, 1 out]
            n273 = Bundle By Name(cluster=w673, "PS_Write"=w672) -> (w671:T20)
            n274 = property on="Tab Control" class="TabCtl (strict)"("Value"=Steptab."PS_WRITE" ("Tab Control")) -> ()  [unwired: 2 in, 2 out]
          }
          frame "READ_DATA" {
            n275 = Unbundle By Name(w681) -> ("READ_DATAS"=w682:T6)
            n276 = Unflatten From String(type=w682, binary string=w683, error in (no error)=w685) -> (value=w678:T6, error out=w684:errorcluster)  [unwired: 2 in, 1 out]
            n277 = Bundle By Name(cluster=w681, "READ_DATAS"=w678) -> (w680:T20)
            n278 = property on="Tab Control" class="TabCtl (strict)"("Value"=Steptab."READ_DATA" ("Tab Control")) -> ()  [unwired: 2 in, 2 out]
          }
          frame "DMM_CONFIG" {
            n279 = Unbundle By Name(w689) -> ("DMM_CONFIG"=w687:T9)
            n280 = Unflatten From String(type=w687, binary string=w691, error in (no error)=w693) -> (value=w686:T9, error out=w692:errorcluster)  [unwired: 2 in, 1 out]
            n281 = Bundle By Name(cluster=w689, "DMM_CONFIG"=w686) -> (w688:T20)
            n282 = property on="Tab Control" class="TabCtl (strict)"("Value"=Steptab."DMM_CONFIG" ("Tab Control")) -> ()  [unwired: 2 in, 2 out]
          }
          frame "DAQ_CONFIG" {
            n283 = Unbundle By Name(w697) -> ("DAQ_Config"=w695:T10)
            n284 = Unflatten From String(type=w695, binary string=w699, error in (no error)=w701) -> (value=w694:T10, error out=w700:errorcluster)  [unwired: 2 in, 1 out]
            n285 = Bundle By Name(cluster=w697, "DAQ_Config"=w694) -> (w696:T20)
            n286 = property on="Tab Control" class="TabCtl (strict)"("Value"=Steptab."DAQ_Config" ("Tab Control")) -> ()  [unwired: 2 in, 2 out]
          }
          frame "PCAN_Read" {
            n287 = Unbundle By Name(w705) -> ("CAN_Read"=w703:T14)
            n288 = Unflatten From String(type=w703, binary string=w707, error in (no error)=w709) -> (value=w702:T14, error out=w708:errorcluster)  [unwired: 2 in, 1 out]
            n289 = Bundle By Name(cluster=w705, "CAN_Read"=w702) -> (w704:T20)
            n290 = property on="Tab Control" class="TabCtl (strict)"("Value"=Steptab."CAN_Read" ("Tab Control")) -> ()  [unwired: 2 in, 2 out]
          }
          frame "PCAN_Write" {
            n291 = Unbundle By Name(w713) -> ("CAN_MSGs_Write"=w711:T11)
            n292 = Unflatten From String(type=w711, binary string=w715, error in (no error)=w717) -> (value=w710:T11, error out=w716:errorcluster)  [unwired: 2 in, 1 out]
            n293 = Bundle By Name(cluster=w713, "CAN_MSGs_Write"=w710) -> (w712:T20)
            n294 = property on="Tab Control" class="TabCtl (strict)"("Value"=Steptab."CAN_Write" ("Tab Control")) -> ()  [unwired: 2 in, 2 out]
          }
          frame "Camera" {
            n295 = Unbundle By Name(w721) -> ("Camera"=w719:T15)
            n296 = Unflatten From String(type=w719, binary string=w723, error in (no error)=w725) -> (value=w718:T15, error out=w724:errorcluster)  [unwired: 2 in, 1 out]
            n297 = Bundle By Name(cluster=w721, "Camera"=w718) -> (w720:T20)
            n298 = property on="Tab Control" class="TabCtl (strict)"("Value"=Steptab."Camera" ("Tab Control")) -> ()  [unwired: 2 in, 2 out]
          }
          frame "MCU_Flashing" {
            n299 = Unbundle By Name(w729) -> ("MCU Flashing"=w730:T17)
            n300 = Unflatten From String(type=w730, binary string=w732, error in (no error)=w733) -> (value=w728:T17, error out=w731:errorcluster)  [unwired: 2 in, 1 out]
            n301 = Bundle By Name(cluster=w729, "MCU Flashing"=w728) -> (w727:T20)
            n302 = property on="Tab Control" class="TabCtl (strict)"("Value"=Steptab."MCU_Flashing" ("Tab Control")) -> ()  [unwired: 2 in, 2 out]
          }
          frame "Noeway_Flashing" {
            n303 = Unbundle By Name(w739) -> ("Noeway_Flashing"=w736:T16)
            n304 = Unflatten From String(type=w736, binary string=w740, error in (no error)=w741) -> (value=w737:T16, error out=w735:errorcluster)  [unwired: 2 in, 1 out]
            n305 = Bundle By Name(cluster=w739, "Noeway_Flashing"=w737) -> (w738:T20)
            n306 = property on="Tab Control" class="TabCtl (strict)"("Value"=Steptab."Noeway_Flashing" ("Tab Control")) -> ()  [unwired: 2 in, 2 out]
          }
          frame "SSL_Certification" {
            n307 = Unbundle By Name(w747) -> ("SSL"=w744:T18)
            n308 = Unflatten From String(type=w744, binary string=w748, error in (no error)=w749) -> (value=w745:T18, error out=w743:errorcluster)  [unwired: 2 in, 1 out]
            n309 = Bundle By Name(cluster=w747, "SSL"=w745) -> (w746:T20)
            n310 = property on="Tab Control" class="TabCtl (strict)"("Value"=Steptab."SSL_Certification" ("Tab Control")) -> ()  [unwired: 2 in, 2 out]
          }
        }
      }
      frame "Save" {
        n311 = Unbundle By Name(w777) -> ("Scripts"=w772:T21[], "Children Symbols"=w771:i32[][], "Parrent Symbol"=w770:i32[], "Configurations:"=w755:string, "Tab Control"=w769:refnum<vi>, "Config"=w754:string)
        n312 = Empty String/Path?(string/path=w754) -> (empty?=w756:bool)
        n313 = call "Specify_Path.vi"("Path_Enum"=enum16{"Find_Path", "Get_Path"}."Get_Path", "error in (no error)"=w778) -> ("Settings"=w759:path, "error out"=w775:errorcluster)  [unwired: 6 in, 6 out]
        n314 = Select(t=w755, s=w756, f=w754) -> (s? t:f=w753:string)
        n315 = Concatenate Strings(w753, ".bin" ("string")) -> (w776:string)
        n316 = Bundle By Name(cluster=T20 {"Script_Tree"=refnum, "Scripts"=[], "ScriptDetails"={"Script Name"="", "Steps"=[]}, "Current Step"={"StepName"="", "StepDetails"="", "Type"=enum."RELAY_CHANNEL_WRITE"}, "ScriptName"="", "StepName"="", "Children Symbols"=[], "Parrent Symbol"=[], "Configurations:"="", "Config"="", "Scriptno."=0, "PS_Write"={"Set_parameter"=0, "VOLTAGE"="", "CURRENT"="", "OUTPUT"=FALSE, "Delay"=FALSE, "Delay time"=0.0}, "DMM_CONFIG"={"CONFIG PARAMETER"=0, "AUTO RANGE"=FALSE, "RANGE"="", "Delay"=FALSE, "Delay time"=0.0}, "READ_DATAS"={"EQUIPMENT"=0, "PARAMETER"=0, "LSL"=0.0, "USL"=0.0, "RESULT"="", "UNIT"="", "Delay"=FALSE, "Delay time"=0.0}, "Set_Channel_Relay"={"Relay_CH_Array"=[]}, "DAQ_Config"={"AUTO RANGE"=FALSE, "CHANNEL LIST"="", "SELECT Card"=0, "SELECT SLOT"=0, "Function"=0}, "CAN_MSGs_Write"={"Scaling Factor"=0, "Physical value"=0.0, "CAN_Frames"={"CAN_ID"=0, "MSGTYPE"=0, "Payload"=[], "Length"=0}, "Offset value"=0.0, "Framing datas"=[], "CAN_Frame Enable"=FALSE, "Add Signal"=FALSE, "Delete Signal"=FALSE, "Signal Values"=[], "Time(ms)"=0.0, "Repetition"=FALSE, "Delay"=FALSE, "Delay time"=0.0}, "CAN_Read"={"Database"="", "Signal"="", "BYTES"=[], "ReadPayload"=[], "String_Data"="", "ReadValue"=0.0, "CANID"=0, "SERVICE ID"=0, "SUB-SERVICE ID"=0, "DELAY "=FALSE, "Delay time(ms)"=0.0}, "Camera"={"Trigger"=FALSE, "Prog No."="", "Delay"=FALSE, "Delay time"=0.0, "Storage"="", "Col no."="", "Row no."=""}, "Tab Control"=refnum, "MCU Flashing"={"Result Path"=path "", "Result"=""}, "Noeway_Flashing"={"Neoway_Firmware"=path "", "RESULT STRING"="", "Delay"=FALSE, "Delay time"=0.0}, "SSL"={"SSL_EXE"=path "", "RESULT STRING"="", "Delay"=FALSE, "Delay time"=0.0}} ("Data Cluster"), "Scripts"=w772, "Children Symbols"=w771, "Parrent Symbol"=w770, "Configurations:"=w755, "Tab Control"=w769) -> (w750:T20)
        n317 = Build Path(base path=w759, name or relative path=w776) -> (appended path=w773:path)
        n318 = Bundle By Name(cluster=w777, "Configurations:"=w755, "Config"="") -> (w758:T20)
        n319 = Flatten To String(anything=w750, error in (no error)=w775) -> (data string=w767:string, error out=w768:errorcluster)  [unwired: 2 in, 1 out]
        n320 = call "BIN_File.vi"("Enum"=enum16{"Read", "Write"}."Write", "error in"=w768, "Data"=w767, "Path"=w773) -> ("error out"=w763:errorcluster)  [unwired: 6 in, 1 out]
        n321 = call "Setting_Screen_Queue_Comm_FGV.vi"("error in (no error)"=w763, "Enum"=Setting_Screen_FGV_Queue_Control."Get") -> ("error Out"=w762:errorcluster, "queue Out"=w765:refnum<queue>)  [unwired: 8 in]
        n322 = call "Setting_Screen_Enqueue Message (Array).vi"("error in (no error)"=w762, "Message Array"=string[] ["ReadSelected"], "Message Queue"=w765) -> ("error out"=w761:errorcluster)  [unwired: 7 in, 1 out]
      }
      frame "SaveAsDisp" {
        n323 = Variant To Data(error in=w813, type="" ("Config"), Variant=w783) -> (data=w779:string, error out=w784:errorcluster)
        n324 = Unbundle By Name(w812) -> ("Scripts"=w806:T21[], "Children Symbols"=w805:i32[][], "Parrent Symbol"=w804:i32[], "Configurations:"=w789:string, "Tab Control"=w803:refnum<vi>, "Config"=w788:string)
        n325 = Empty String/Path?(string/path=w788) -> (empty?=w790:bool)
        n326 = property on="Configurations:" class="CmbBox"() -> ("Strings[]"=w781:string[])  [unwired: 2 in, 2 out]
        n327 = Select(t=w789, s=w790, f=w788) -> ()  [unwired: 1 out]
        n328 = Build Array (concatenate)(w781, w779) -> (w780:string[])
        n329 = call "Specify_Path.vi"("Path_Enum"=enum16{"Find_Path", "Get_Path"}."Get_Path", "error in (no error)"=w784) -> ("Settings"=w793:path, "error out"=w810:errorcluster)  [unwired: 6 in, 6 out]
        n330 = Bundle By Name(cluster=T20 {"Script_Tree"=refnum, "Scripts"=[], "ScriptDetails"={"Script Name"="", "Steps"=[]}, "Current Step"={"StepName"="", "StepDetails"="", "Type"=enum."RELAY_CHANNEL_WRITE"}, "ScriptName"="", "StepName"="", "Children Symbols"=[], "Parrent Symbol"=[], "Configurations:"="", "Config"="", "Scriptno."=0, "PS_Write"={"Set_parameter"=0, "VOLTAGE"="", "CURRENT"="", "OUTPUT"=FALSE, "Delay"=FALSE, "Delay time"=0.0}, "DMM_CONFIG"={"CONFIG PARAMETER"=0, "AUTO RANGE"=FALSE, "RANGE"="", "Delay"=FALSE, "Delay time"=0.0}, "READ_DATAS"={"EQUIPMENT"=0, "PARAMETER"=0, "LSL"=0.0, "USL"=0.0, "RESULT"="", "UNIT"="", "Delay"=FALSE, "Delay time"=0.0}, "Set_Channel_Relay"={"Relay_CH_Array"=[]}, "DAQ_Config"={"AUTO RANGE"=FALSE, "CHANNEL LIST"="", "SELECT Card"=0, "SELECT SLOT"=0, "Function"=0}, "CAN_MSGs_Write"={"Scaling Factor"=0, "Physical value"=0.0, "CAN_Frames"={"CAN_ID"=0, "MSGTYPE"=0, "Payload"=[], "Length"=0}, "Offset value"=0.0, "Framing datas"=[], "CAN_Frame Enable"=FALSE, "Add Signal"=FALSE, "Delete Signal"=FALSE, "Signal Values"=[], "Time(ms)"=0.0, "Repetition"=FALSE, "Delay"=FALSE, "Delay time"=0.0}, "CAN_Read"={"Database"="", "Signal"="", "BYTES"=[], "ReadPayload"=[], "String_Data"="", "ReadValue"=0.0, "CANID"=0, "SERVICE ID"=0, "SUB-SERVICE ID"=0, "DELAY "=FALSE, "Delay time(ms)"=0.0}, "Camera"={"Trigger"=FALSE, "Prog No."="", "Delay"=FALSE, "Delay time"=0.0, "Storage"="", "Col no."="", "Row no."=""}, "Tab Control"=refnum, "MCU Flashing"={"Result Path"=path "", "Result"=""}, "Noeway_Flashing"={"Neoway_Firmware"=path "", "RESULT STRING"="", "Delay"=FALSE, "Delay time"=0.0}, "SSL"={"SSL_EXE"=path "", "RESULT STRING"="", "Delay"=FALSE, "Delay time"=0.0}} ("Data Cluster"), "Scripts"=w806, "Children Symbols"=w805, "Parrent Symbol"=w804, "Configurations:"=w779, "Tab Control"=w803) -> (w801:T20)
        n331 = Concatenate Strings(w779, ".bin" ("string")) -> (w811:string)
        n332 = property on="Configurations:" class="CmbBox"("Strings[]"=w780, "Value"=w779) -> ()  [unwired: 2 in, 2 out]
        n333 = Build Path(base path=w793, name or relative path=w811) -> (appended path=w808:path)
        n334 = Bundle By Name(cluster=w812, "Configurations:"=w779, "Config"="") -> (w792:T20)
        n335 = Flatten To String(anything=w801, error in (no error)=w810) -> (data string=w800:string, error out=w802:errorcluster)  [unwired: 2 in, 1 out]
        n336 = call "BIN_File.vi"("Enum"=enum16{"Read", "Write"}."Write", "error in"=w802, "Data"=w800, "Path"=w808) -> ("error out"=w786:errorcluster)  [unwired: 6 in, 1 out]
        n337 = flat-sequence {
          tunnel: w786 -> [w816]
          tunnel: [w815] -> w785
          frame #0 {
            n338 = property on="SaveAs Name:" class="Str"(error in=w816, "Visible"=FALSE, "Value"="" ("SaveAs Name:")) -> (error out=w815:errorcluster)  [unwired: 1 in, 1 out]
          }
        }
        n339 = call "Setting_Screen_Queue_Comm_FGV.vi"("error in (no error)"=w785, "Enum"=Setting_Screen_FGV_Queue_Control."Get") -> ("error Out"=w796:errorcluster, "queue Out"=w798:refnum<queue>)  [unwired: 8 in]
        n340 = call "Setting_Screen_Enqueue Message (Array).vi"("error in (no error)"=w796, "Message Array"=string[] ["ReadSelected"], "Message Queue"=w798) -> ("error out"=w795:errorcluster)  [unwired: 7 in, 1 out]
      }
      frame "SaveAs" {
        n341 = flat-sequence {
          tunnel: w819 -> [w824]
          tunnel: [w823] -> w818
          frame #0 {
            n342 = property on="SaveAs Name:" class="Str"(error in=w824, "Visible"=TRUE, "Value"="" ("SaveAs Name:")) -> (error out=w823:errorcluster)  [unwired: 1 in, 1 out]
          }
        }
      }
      frame "NewConfig" {
        w828 = ""
        n343 = Variant To Data(error in=w844, type="", Variant=w841) -> (data=w826:string, error out=w837:errorcluster)
        n344 = property on="Configurations:" class="CmbBox"() -> ("Strings[]"=w827:string[])  [unwired: 2 in, 2 out]
        n345 = Build Array (concatenate)(w827, w826) -> (w825:string[])
        n346 = Bundle By Name(cluster=w845, "ScriptName"=w828, "StepName"=w828, "Children Symbols"=i32[][] [], "Parrent Symbol"=i32[] [], "Current Step"=T22 {"StepName"="", "StepDetails"="", "Type"=enum."RELAY_CHANNEL_WRITE"}, "ScriptDetails"=T21 {"Script Name"="", "Steps"=[]}, "Scripts"=T21[] [{"Script Name"="", "Steps"=[{"StepName"="", "StepDetails"="", "Type"=enum."RELAY_CHANNEL_WRITE"}]}], "Config"=w826) -> (w840:T20)
        n347 = property on="Configurations:" class="CmbBox"("Strings[]"=w825) -> ()  [unwired: 2 in, 2 out]
        n348 = call "Setting_Screen_Queue_Comm_FGV.vi"("error in (no error)"=w837, "Enum"=Setting_Screen_FGV_Queue_Control."Get") -> ("error Out"=w836:errorcluster, "queue Out"=w839:refnum<queue>)  [unwired: 8 in]
        n349 = call "Setting_Screen_Enqueue Message (Array).vi"("error in (no error)"=w836, "Message Array"=string[] ["Reset Step", "Update Display"], "Message Queue"=w839) -> ("error out"=w835:errorcluster)  [unwired: 7 in, 1 out]
        n350 = flat-sequence {
          tunnel: w835 -> [w849]
          tunnel: [w848] -> w843
          frame #0 {
            w846 = ""
            n351 = local write "Script_Tree"(w846) -> ()
            n352 = property on="New_Config_name" class="Str"(error in=w849, "Visible"=FALSE, "Value"=w846) -> (error out=w848:errorcluster)  [unwired: 1 in, 1 out]
          }
        }
      }
      frame "NewConfigDisp" {
        n353 = flat-sequence {
          tunnel: w851 -> [w856]
          tunnel: [w855] -> w850
          frame #0 {
            n354 = property on="New_Config_name" class="Str"(error in=w856, "Visible"=TRUE, "Value"="" ("New_Config_name")) -> (error out=w855:errorcluster)  [unwired: 1 in, 1 out]
          }
        }
      }
      frame "INSTR_CONFIG" {
        n355 = Unbundle By Name(w858) -> ("Configurations:"=w857:string)
        n356 = call "Instr Config.vi"("error constant"=w860, "Configuration"=w857) -> ("error out"=w859:errorcluster)  [unwired: 9 in]
      }
      frame "Stepname" {
        n357 = Variant To Data(error in=w867, type="", Variant=w863) -> (data=w861:string, error out=w865:errorcluster)
        n358 = Bundle By Name(cluster=w866, "Current Step.StepName"=w861, "StepName"=w861) -> (w862:T20)
      }
      frame "Scriptname" {
        n359 = Variant To Data(error in=w874, type="", Variant=w870) -> (data=w868:string, error out=w872:errorcluster)
        n360 = Bundle By Name(cluster=w873, "ScriptName"=w868) -> (w869:T20)
      }
      frame "Update Display" {
        # "Update The Display according to the tree ."
        n361 = Unbundle By Name(w889) -> ("SSL"=w875:T18, "Noeway_Flashing"=w876:T16, "MCU Flashing"=w877:T17, "Set_Channel_Relay"=w883:T2, "PS_Write"=w886:T4, "ScriptName"=w887:string, "StepName"=w888:string, "DMM_CONFIG"=w885:T9, "READ_DATAS"=w884:T6, "CAN_MSGs_Write"=w881:T11, "CAN_Read"=w882:T14, "DAQ_Config"=w879:T10, "Camera"=w878:T15)
        n362 = To Variant(anything=w881) -> (Variant=w880:variant)
        n363 = local write "Set_Channel_Relay"(w883) -> ()
        n364 = local write "MCU Flashing"(w877) -> ()
        n365 = local write "PS_Write"(w886) -> ()
        n366 = local write "Script Name"(w887) -> ()
        n367 = local write "Step Name"(w888) -> ()
        n368 = property on="CAN_MSGs_Write" class="Clust"("Value"=w880) -> ()  [unwired: 2 in, 2 out]
        n369 = property on="CAN_Read" class="Clust (strict)"("Value"=w882) -> ()  [unwired: 2 in, 2 out]
        n370 = local write "DMM_CONFIG"(w885) -> ()
        n371 = local write "READ_DATAS"(w884) -> ()
        n372 = local write "Noeway_Flashing"(w876) -> ()
        n373 = local write "SSL"(w875) -> ()
        n374 = local write "DAQ_Config"(w879) -> ()
        n375 = local write "Camera"(w878) -> ()
        n376 = Merge Errors(w890) -> (w891:errorcluster)
      }
      frame "Error" {
        # "Error - Display an error dialog. This message is sent by the \"Error Handler\" VIs at the end of other loops in this application."
        n377 = Variant To Data(error in=w898, type=errorcluster {"status"=FALSE, "code"=0, "source"=""} ("error constant"), Variant=w896) -> (data=w894:errorcluster, error out=w893:errorcluster)
        n378 = call <vilib>:"Simple Error Handler.vi"("error in (no error)"=w894) -> ()  [unwired: 4 in, 5 out]
        n379 = Merge Errors(w893) -> (w892:errorcluster)
      }
      frame "Confirm Quit" {
        # "Confirm Quit - Message that can confirm whether or not the user wants to exit the application."
        n380 = call "Setting_Screen_Enque_Message_FGV.vi"("Priority"=TRUE ("Priority Message? (F)"), "error in (no error)"=w901, "Message"="Exit") -> ("error out"=w902:errorcluster)  [unwired: 8 in]
        n381 = Merge Errors(w902) -> (w903:errorcluster)
      }
      frame "Exit" {
        # "Exit - Exit the application."
        n382 = Variant To Data(type=errorcluster {"status"=FALSE, "code"=0, "source"=""} ("error constant"), Variant=w911) -> (data=w912:errorcluster)  [unwired: 1 in, 1 out]
        n383 = call <vilib>:"Simple Error Handler.vi"("error in (no error)"=w912) -> ()  [unwired: 4 in, 5 out]
        n384 = call "Setting_Screen_Queue_Comm_FGV.vi"("error in (no error)"=w909, "Enum"=Setting_Screen_FGV_Queue_Control."Release") -> ("error Out"=w908:errorcluster)  [unwired: 8 in, 1 out]
        n385 = call "Fire User Event - Stop.vi"("User Event - Stop"=w907) -> ("error out"=w905:errorcluster)  [unwired: 10 in]
        n386 = call "Fire User Event - Stop.vi"("User Event - Stop"=w914) -> ("error out"=w906:errorcluster)  [unwired: 10 in]
        n387 = Merge Errors(w906, w905, w908) -> (w915:errorcluster)
      }
      frame Default {
        # "'Default' case only runs if there is a message that isn't defined in any of the other cases.  Output a programming error."
        n388 = xnode "Error Ring"("parameter 0"=w918) -> ("error out"=w919:errorcluster)
      }
    }
    n389 = call "Setting_Screen_Error_Handler_MHL_FGV.vi"("error in (no error)"=w30) -> ("error Out"=w29:errorcluster)  [unwired: 10 in]
  }
  n390 = while {
    shift-right: [w931] -> w21
    shift-left: w18 -> [w932]
    tunnel: [w928] -> w19
    stop <- w930 stop-if-true
    # "Event Handling Loop"
    n391 = event shown="[27] \"Configurations:\": Value Change" {
      selector: w932 -> [_ _ _ _ _ _ _ _ _ _ _ _ _ _ _ _ _ _ _ _ _ _ _ _ _ _ _ _ _ _ _ _ _ _ _ _ _ _ _ _]
      dyn-events: [_ _ _ _ _ _ _ _ _ _ _ _ _ _ _ _ _ _ _ _ _ _ _ _ _ _ _ _ _ _ _ _ _ _ _ _ _ _ _ _] -> w931
      timeout: _ -> [_ _ _ _ _ _ _ _ _ _ _ _ _ _ _ _ _ _ _ _ _ _ _ _ _ _ _ _ _ _ _ _ _ _ _ _ _ _ _ _]
      tunnel: [_ _ _ _ _ _ _ _ _ _ _ _ _ _ _ _ _ _ _ _ _ _ _ _ _ _ _ _ _ _ _ _ _ _ _ _ _ TRUE ("Discard?") _ _] -> w930
      tunnel: [w934 w936 w939 w942 w945 w948 w951 w954 w957 w960 w965 w970 w975 w980 w985 w992 w995 w1000 w1004 w1008 w1014 w1017 w1022 w1023 w1026 w1031 w1034 w1038 w1041 w1046 w1051 w1055 w1059 w1062 w1067 _ w1071 _ w1075 w1078] -> w929
      event "New Script": Value Change {
        n392 = event-data() -> ()  [unwired: 1 in, 1 out]
        n393 = call "Setting_Screen_Enque_Message_FGV.vi"("Priority"=TRUE ("Priority Message? (F)"), "Message"="NewScript") -> ("error out"=w934:errorcluster)  [unwired: 9 in]
      }
      event "New Step": Value Change {
        n394 = event-data() -> ()  [unwired: 1 in, 1 out]
        n395 = call "Setting_Screen_Enque_Message_FGV.vi"("Priority"=TRUE ("Priority Message? (F)"), "Message"="NewStep") -> ("error out"=w936:errorcluster)  [unwired: 9 in]
      }
      event "UpdateStep": Value Change {
        n396 = event-data() -> ()  [unwired: 1 in, 1 out]
        n397 = call "Setting_Screen_Enque_Message_FGV.vi"("Priority"=TRUE ("Priority Message? (F)"), "Message"="UpdateStep") -> ("error out"=w939:errorcluster)  [unwired: 9 in]
      }
      event "Add Script": Value Change {
        n398 = event-data() -> ()  [unwired: 1 in, 1 out]
        n399 = call "Setting_Screen_Enque_Message_FGV.vi"("Priority"=TRUE ("Priority Message? (F)"), "Message"="AddScript") -> ("error out"=w942:errorcluster)  [unwired: 9 in]
      }
      event "ADD NEXT SCRIPT": Value Change {
        n400 = event-data() -> ()  [unwired: 1 in, 1 out]
        n401 = call "Setting_Screen_Enque_Message_FGV.vi"("Priority"=TRUE ("Priority Message? (F)"), "Message"="AddnextScript") -> ("error out"=w945:errorcluster)  [unwired: 9 in]
      }
      event "STEP_UP": Value Change {
        n402 = event-data() -> ()  [unwired: 1 in, 1 out]
        n403 = call "Setting_Screen_Enque_Message_FGV.vi"("Priority"=TRUE ("Priority Message? (F)"), "Message"="Step_up") -> ("error out"=w948:errorcluster)  [unwired: 9 in]
      }
      event "STEP_DOWN": Value Change {
        n404 = event-data() -> ()  [unwired: 1 in, 1 out]
        n405 = call "Setting_Screen_Enque_Message_FGV.vi"("Priority"=TRUE ("Priority Message? (F)"), "Message"="Step_down") -> ("error out"=w951:errorcluster)  [unwired: 9 in]
      }
      event "Add Step": Value Change {
        n406 = event-data() -> ()  [unwired: 1 in, 1 out]
        n407 = call "Setting_Screen_Enque_Message_FGV.vi"("Priority"=TRUE ("Priority Message? (F)"), "Message"="AddStep") -> ("error out"=w954:errorcluster)  [unwired: 9 in]
      }
      event "Delete Script": Value Change {
        n408 = event-data() -> ()  [unwired: 1 in, 1 out]
        n409 = call "Setting_Screen_Enque_Message_FGV.vi"("Priority"=TRUE ("Priority Message? (F)"), "Message"="DelScript") -> ("error out"=w957:errorcluster)  [unwired: 9 in]
      }
      event "Delete Step": Value Change {
        n410 = event-data() -> ()  [unwired: 1 in, 1 out]
        n411 = call "Setting_Screen_Enque_Message_FGV.vi"("Priority"=TRUE ("Priority Message? (F)"), "Message"="DelStep") -> ("error out"=w960:errorcluster)  [unwired: 9 in]
      }
      event Value Change {
        n412 = event-data() -> ()  [unwired: 1 in, 1 out]
        n413 = To Variant(anything="Set_Channel_Relay") -> (Variant=w964:variant)
        n414 = call "Setting_Screen_Enque_Message_FGV.vi"("Priority"=TRUE ("Priority Message? (F)"), "Message Data"=w964, "Message"="Relay_Channel_Write") -> ("error out"=w965:errorcluster)  [unwired: 8 in]
      }
      event Value Change {
        n415 = event-data() -> ()  [unwired: 1 in, 1 out]
        n416 = To Variant(anything="DMM_CONFIG") -> (Variant=w968:variant)
        n417 = call "Setting_Screen_Enque_Message_FGV.vi"("Priority"=TRUE ("Priority Message? (F)"), "Message Data"=w968, "Message"="DMM_CONFIG") -> ("error out"=w970:errorcluster)  [unwired: 8 in]
      }
      event Value Change {
        n418 = event-data() -> ()  [unwired: 1 in, 1 out]
        n419 = To Variant(anything="DAQ_Config") -> (Variant=w974:variant)
        n420 = call "Setting_Screen_Enque_Message_FGV.vi"("Priority"=TRUE ("Priority Message? (F)"), "Message Data"=w974, "Message"="DAQ_CONFIG") -> ("error out"=w975:errorcluster)  [unwired: 8 in]
      }
      event Value Change {
        n421 = event-data() -> ()  [unwired: 1 in, 1 out]
        n422 = To Variant(anything="READ_DATAS") -> (Variant=w978:variant)
        n423 = call "Setting_Screen_Enque_Message_FGV.vi"("Priority"=TRUE ("Priority Message? (F)"), "Message Data"=w978, "Message"="READ_DATAS") -> ("error out"=w980:errorcluster)  [unwired: 8 in]
      }
      event Value Change {
        n424 = event-data() -> ()  [unwired: 1 in, 1 out]
        n425 = To Variant(anything="PS_Write") -> (Variant=w984:variant)
        n426 = call "Setting_Screen_Enque_Message_FGV.vi"("Priority"=TRUE ("Priority Message? (F)"), "Message Data"=w984, "Message"="PS_WRITE") -> ("error out"=w985:errorcluster)  [unwired: 8 in]
      }
      event Value Change {
        n427 = event-data() -> ()  [unwired: 1 in, 1 out]
        n428 = To Variant(anything="CAN_Read") -> (Variant=w988:variant)
        n429 = call "Setting_Screen_Enque_Message_FGV.vi"("Priority"=TRUE, "Message Data"=w988, "Message"="CAN_Read") -> ("error out"=w992:errorcluster)  [unwired: 8 in]
      }
      event Value Change {
        n430 = event-data() -> ()  [unwired: 1 in, 1 out]
        n431 = To Variant(anything="MCU Flashing") -> (Variant=w993:variant)
        n432 = call "Setting_Screen_Enque_Message_FGV.vi"("Priority"=TRUE, "Message Data"=w993, "Message"="MCU_Flashing") -> ("error out"=w995:errorcluster)  [unwired: 8 in]
      }
      event Value Change {
        n433 = event-data() -> ()  [unwired: 1 in, 1 out]
        n434 = To Variant(anything="Noeway_Flashing") -> (Variant=w998:variant)
        n435 = call "Setting_Screen_Enque_Message_FGV.vi"("Priority"=TRUE, "Message Data"=w998, "Message"="Neoway") -> ("error out"=w1000:errorcluster)  [unwired: 8 in]
      }
      event Value Change {
        n436 = event-data() -> ()  [unwired: 1 in, 1 out]
        n437 = To Variant(anything="SSL") -> (Variant=w1005:variant)
        n438 = call "Setting_Screen_Enque_Message_FGV.vi"("Priority"=TRUE, "Message Data"=w1005, "Message"="SSL") -> ("error out"=w1004:errorcluster)  [unwired: 8 in]
      }
      event Value Change {
        n439 = event-data() -> ()  [unwired: 1 in, 1 out]
        n440 = call "Setting_Screen_Enque_Message_FGV.vi"("Priority"=TRUE, "Message Data"="CAN_MSGs_Write", "Message"="CAN_Write") -> ("error out"=w1008:errorcluster)  [unwired: 8 in]
      }
      event Value Change {
        n441 = event-data() -> ()  [unwired: 1 in, 1 out]
        n442 = call "Setting_Screen_Enque_Message_FGV.vi"("Priority"=TRUE, "Message"="Add_Signal") -> ("error out"=w1014:errorcluster)  [unwired: 9 in]
      }
      event Value Change {
        n443 = event-data() -> ()  [unwired: 1 in, 1 out]
        n444 = call "Setting_Screen_Enque_Message_FGV.vi"("Priority"=TRUE, "Message"="Delete_Signal") -> ("error out"=w1017:errorcluster)  [unwired: 9 in]
      }
      event Value Change {
        n445 = event-data() -> ()  [unwired: 1 in, 1 out]
        n446 = To Variant(anything="Camera") -> (Variant=w1019:variant)
        n447 = call "Setting_Screen_Enque_Message_FGV.vi"("Priority"=TRUE, "Message Data"=w1019, "Message"="Camera") -> ("error out"=w1022:errorcluster)  [unwired: 8 in]
      }
      event "Save": Value Change {
        n448 = event-data() -> ()  [unwired: 1 in, 1 out]
        n449 = call "Setting_Screen_Enque_Message_FGV.vi"("Priority"=TRUE ("Priority Message? (F)"), "Message"="Save") -> ("error out"=w1023:errorcluster)  [unwired: 9 in]
      }
      event "Save As": Value Change {
        n450 = event-data() -> ()  [unwired: 1 in, 1 out]
        n451 = call "Setting_Screen_Enque_Message_FGV.vi"("Priority"=TRUE ("Priority Message? (F)"), "Message"="SaveAs") -> ("error out"=w1026:errorcluster)  [unwired: 9 in]
      }
      event "SaveAs Name:": Value Change {
        n452 = event-data() -> ()  [unwired: 1 in, 1 out]
        n453 = To Variant(anything="SaveAs Name:") -> (Variant=w1029:variant)
        n454 = call "Setting_Screen_Enque_Message_FGV.vi"("Priority"=TRUE ("Priority Message? (F)"), "Message Data"=w1029, "Message"="SaveAsDisp") -> ("error out"=w1031:errorcluster)  [unwired: 8 in]
      }
      event "New Config": Value Change {
        n455 = event-data() -> ()  [unwired: 1 in, 1 out]
        n456 = call "Setting_Screen_Enque_Message_FGV.vi"("Priority"=TRUE ("Priority Message? (F)"), "Message"="NewConfigDisp") -> ("error out"=w1034:errorcluster)  [unwired: 9 in]
      }
      event "Configurations:": Value Change {
        n457 = event-data() -> ()  [unwired: 1 in, 1 out]
        n458 = call "Setting_Screen_Enque_Message_FGV.vi"("Priority"=TRUE ("Priority Message? (F)"), "Message Data"="Configurations:", "Message"="ReadSelected") -> ("error out"=w1038:errorcluster)  [unwired: 8 in]
      }
      event "Instr.": Value Change {
        n459 = event-data() -> ()  [unwired: 1 in, 1 out]
        n460 = call "Setting_Screen_Enque_Message_FGV.vi"("Priority"=TRUE ("Priority Message? (F)"), "Message"="INSTR_CONFIG") -> ("error out"=w1041:errorcluster)  [unwired: 9 in]
      }
      event "Step Name": Value Change {
        n461 = event-data() -> ()  [unwired: 1 in, 1 out]
        n462 = To Variant(anything="Step Name") -> (Variant=w1044:variant)
        n463 = call "Setting_Screen_Enque_Message_FGV.vi"("Priority"=TRUE ("Priority Message? (F)"), "Message Data"=w1044, "Message"="Stepname") -> ("error out"=w1046:errorcluster)  [unwired: 8 in]
      }
      event "Script Name": Value Change {
        n464 = event-data() -> ()  [unwired: 1 in, 1 out]
        n465 = To Variant(anything="Script Name") -> (Variant=w1050:variant)
        n466 = call "Setting_Screen_Enque_Message_FGV.vi"("Priority"=TRUE ("Priority Message? (F)"), "Message Data"=w1050, "Message"="Scriptname") -> ("error out"=w1051:errorcluster)  [unwired: 8 in]
      }
      event "New_Config_name": Value Change {
        n467 = event-data() -> ()  [unwired: 1 in, 1 out]
        n468 = call "Setting_Screen_Enque_Message_FGV.vi"("Priority"=TRUE ("Priority Message? (F)"), "Message Data"="New_Config_name", "Message"="NewConfig") -> ("error out"=w1055:errorcluster)  [unwired: 8 in]
      }
      event "New Step Name": Value Change {
        n469 = event-data() -> ()  [unwired: 1 in, 2 out]
        n470 = call "Setting_Screen_Enque_Message_FGV.vi"("Priority"=TRUE ("Priority Message? (F)"), "Message Data"="New Step Name", "Message"="NewStepname") -> ("error out"=w1059:errorcluster)  [unwired: 8 in]
      }
      event "Rename Step": Value Change {
        n471 = event-data() -> ()  [unwired: 1 in, 2 out]
        n472 = call "Setting_Screen_Enque_Message_FGV.vi"("Priority"=TRUE ("Priority Message? (F)"), "Message"="Rename_Step") -> ("error out"=w1062:errorcluster)  [unwired: 9 in]
      }
      event Panel Close? {
        n473 = event-data() -> ()  [unwired: 1 in, 1 out]
        n474 = call "Setting_Screen_Enque_Message_FGV.vi"("Priority"=TRUE ("Priority Message? (F)"), "Message"="Confirm Quit") -> ("error out"=w1067:errorcluster)  [unwired: 9 in]
        n475 = event-data("Discard?"=TRUE) -> ()  [unwired: 1 in, 1 out]
      }
      event Application Instance Close {
        n476 = event-data() -> ()  [unwired: 1 in, 1 out]
      }
      event "Exit": Value Change {
        n477 = event-data() -> ()  [unwired: 1 in, 1 out]
        n478 = call "Setting_Screen_Enque_Message_FGV.vi"("Priority"=TRUE ("Priority Message? (F)"), "Message"="Exit") -> ("error out"=w1071:errorcluster)  [unwired: 9 in]
      }
      event User Event {
        (unwired) "\"Exit\" button pressed" ("VI Stopped")
        n479 = event-data() -> ()  [unwired: 1 in, 1 out]
      }
      event "Script_Tree": Value Change {
        n480 = event-data() -> ()  [unwired: 1 in, 4 out]
        n481 = To Variant(anything="Script_Tree") -> (Variant=w1074:variant)
        n482 = call "Setting_Screen_Enque_Message_FGV.vi"("Priority"=TRUE ("Priority Message? (F)"), "Message Data"=w1074, "Message"="ScriptTree") -> ("error out"=w1075:errorcluster)  [unwired: 8 in]
      }
      event "Script_Tree": Shortcut Menu Selection (User) {
        n483 = event-data() -> ("ItemTag"=w1079:string)  [unwired: 1 in]
        n484 = case shown="\"En/Disable_Script\"" w1079 {
          tunnel: [_ w1082] -> w1078
          frame Default {
          }
          frame "En/Disable_Script" {
            n485 = call "Setting_Screen_Enque_Message_FGV.vi"("Priority"=TRUE, "Message"="En/Dis_Script") -> ("error out"=w1082:errorcluster)  [unwired: 9 in]
          }
        }
      }
    }
    n486 = call "Setting_Screen_Error_Handler_EHL_FGV.vi"("error in (no error)"=w929) -> ("error Out"=w928:errorcluster)  [unwired: 10 in]
  }
  n487 = Unregister For Events(event registration refnum=w21, error in=w19) -> (error out=w22:errorcluster)
  n488 = Merge Errors(w22, w25) -> (w23:errorcluster)
  n489 = call "Destroy User Event - Stop.vi"("error in (no error)"=w23, "User Event - Stop"=w3) -> ("error out"=w12:errorcluster)  [unwired: 9 in]
  n490 = call <vilib>:"Clear Errors.vi"("error in (no error)"=w12) -> ("error out"=w2:errorcluster)  [unwired: 5 in, 1 out]
  n491 = disable-structure shown="Disabled" {
    disable-tunnel: w2 -> [w1088 _]
    disable-tunnel: [w1086 _] -> w1
    frame Disabled {
      n492 = vi-ref "Launcher_DTU.lvlib:MainLauncher.vi"() -> (w1084:refnum<vi>)
      n493 = invoke class="VI" method="FP.Open"(reference=w1084, error in=w1088, "State"=T27."Standard") -> (error out=w1087:errorcluster)  [unwired: 2 in, 4 out]
      n494 = control-ref of="This VI"() -> (w1085:refnum<vi>)
      n495 = invoke class="VI" method="FP.Close"(reference=w1085, error in=w1087) -> (error out=w1086:errorcluster)  [unwired: 1 in, 2 out]
    }
    frame Enabled {
    }
  }
  "error in (out)" <- w1
